vi "Main.vi"() -> ()   [LabVIEW 2020]
uses:
  Archiv/2022-07-15 Labview Burst Preassure Measuring System_neu/Computer/Controls/IMAQdx.ctl
  Controls/SM_UserInterface.ctl
  Controls/SM_DataLog.ctl
  <vilib>/Platform/TimedLoop/XDataNode/timing_clust.ctl
  <vilib>/Platform/TimedLoop/XDataNode/nitl_modes.ctl
  <vilib>/Platform/TimedLoop/XDataNode/wakeup.ctl
  <vilib>/Analysis/baseanly.llb/Mean (DBL).vi
  <vilib>/platform/TimedLoop/XDataNode/XDataNode.xnode
  <vilib>/ptbypt/NI_PtbyPt.lvlib
  <vilib>/Platform/TimedLoop/XDataNode/XDNodeRunTimeDep.lvlib
  Library/Data Buffer.lvlib
  <vilib>/Analysis/NI_AALBase.lvlib
panel:
  in  "OK Exp 2":bool
  in  "Experiment Comment":string
  in  "Buffer Cam4":T1
  in  "Buffer Cam3":T1
  in  "Buffer Cam2":T1
  in  "Buffer Cam1":T1
  out "LoopTimer Cam3":T2
  out "WriteSpeed Cam3":T3 {"WriteSpeed Worker5" format="%_19f"; "WriteSpeed Worker4" format="%_19f"; "WriteSpeed Worker3" format="%_19f"; "WriteSpeed Worker2" format="%_19f"; "WriteSpeed Worker1" format="%_19f"}
  out "Frames Cam3":T4
  out "LoopTimer Cam4":T2
  out "WriteSpeed Cam4":T3 {"WriteSpeed Worker5" format="%_19f"; "WriteSpeed Worker4" format="%_19f"; "WriteSpeed Worker3" format="%_19f"; "WriteSpeed Worker2" format="%_19f"; "WriteSpeed Worker1" format="%_19f"}
  out "Frames Cam4":T4
  out "LoopTimer Cam2":T2
  out "WriteSpeed Cam2":T3 {"WriteSpeed Worker5" format="%_19f"; "WriteSpeed Worker4" format="%_19f"; "WriteSpeed Worker3" format="%_19f"; "WriteSpeed Worker2" format="%_19f"; "WriteSpeed Worker1" format="%_19f"}
  out "Frames Cam2":T4
  out "Frames Cam1":T4
  out "WriteSpeed Cam1":T3 {"WriteSpeed Worker5" format="%_19f"; "WriteSpeed Worker4" format="%_19f"; "WriteSpeed Worker3" format="%_19f"; "WriteSpeed Worker2" format="%_19f"; "WriteSpeed Worker1" format="%_19f"}
  out "LoopTimer Cam1":T2
  in  "Developer":bool
  out "DataFile":bool
  out "Cam4 Time":string
  out "Cam3 Time":string
  out "Cam2 Time":string
  out "Cam1 Time":string
  in  "OK Exp":bool
  out "Stop":bool
  in  "Experiment Comment":string
  in  "Flow Rate Level":i32 min=0 max=99 step=1
  out "IncLoop DataLog":i32
  out "Pressure (mmHg)":dbl format="%.1f"
  out "Waveform Pressure Cluster":waveform(dbl)[](graph)
  out "meanPressureArray":dbl[](array[numeric])
  out "meanPressure":dbl format="%0.2f"
  out "Camera 4":T5(plugin-control)
  out "StartPressure (mmHg)":dbl format="%.2f"
  out "LogFolder":path
  out "StateDataLog":T6
  out "StateUI":T7
  out "CamInput":bool
  out "Start_DateTime":string
  out "LoopTimer UI":u32
  out "Temp (C)":dbl format="%#.1f"
  out "Waveform Chart Temp":waveform(dbl)(graph)
  out "Status Camera 4":bool
  out "Status Camera 3":bool
  out "Status Camera 2":bool
  out "Status Camera 1":bool
  out "Status Temp. Sensor":bool
  out "Status Pressure Sensor":bool
  in  "User":string
  in  "Experiment Infos":string
  in  "Bursting Mode":string(combo)
  out "ExpTime_ms":i32
  out "ActualTime_ms":i32
  out "Camera 1":T5(plugin-control)
  out "Camera 2":T5(plugin-control)
  out "Camera 3":T5(plugin-control)
  in  "IMAQdxChannel 1":T8="cam0" caption="Camera Channel 1"
  in  "OK Input":bool
  in  "IMAQdxChannel 2":T8="cam0" caption="Camera Channel 2"
  in  "IMAQdxChannel 3":T8="cam0" caption="Camera Channel 3"
  in  "IMAQdxChannel 4":T8="cam0" caption="Camera Channel 4"
  out "Status":string="Video OFF"
  in  "Folder":path=path "C:/Users/Public/Downloads" caption="Select path to store video"
  in  "File Name":string
  in  "OK File":bool
  in  "StartRecord":bool caption="Save Video"
  in  "StopRecord":bool
  out "Pressure Temp (C)":dbl
  out "error out":errorcluster
  in  "Cancel":bool
  # "MRI   TUM"
  # "Burst Pressure Measuring System"
  # "1. Select USB Camera Channel"
  # "Pressure in mmHg"
  # "2. Set the Storage Location & Experiment Data"
  # "Temperature in °C"
  # "3. Video and Data Recording"
  # "Sensor Status"
  # "Set before Start Video"
  # "Set before Start Video"
  # "Set before Start Video"
  # "Set before Start Video"
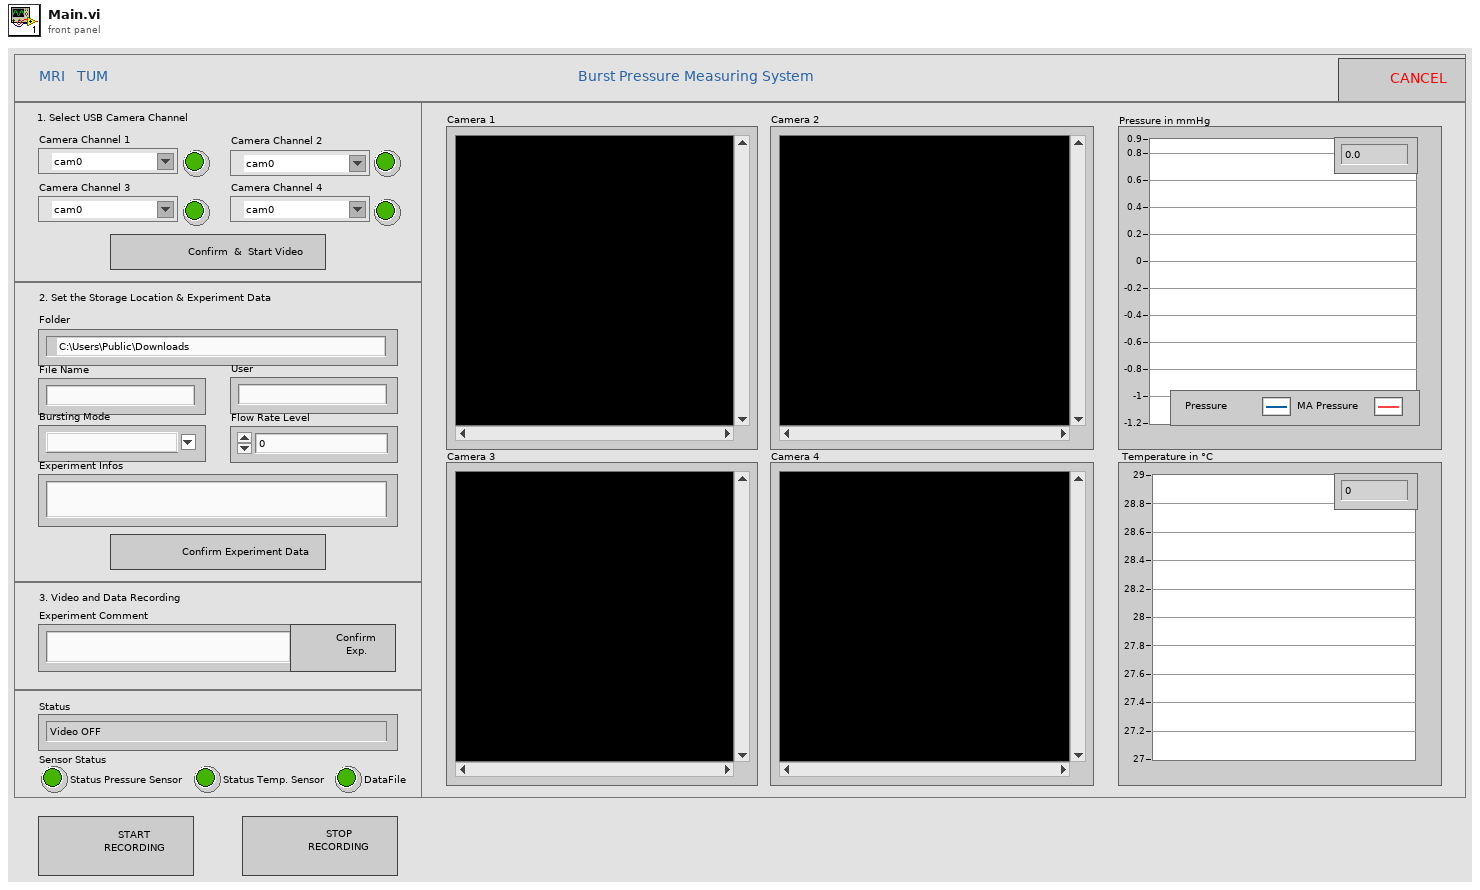
[diagram p1: front panel]
types:
  T1 = cluster{"Skip Count":u32, "Number of Workers":u8, "Number of Images":i32}
  T2 = cluster{"LoopTimerAcqu":u32, "LoopTimer Worker1":u32, "LoopTimer Worker2":u32, "LoopTimer Worker3":u32, "LoopTimer Worker4":u32, "LoopTimer Worker5":u32}
  T3 = cluster{"WriteSpeed Worker1":dbl, "WriteSpeed Worker2":dbl, "WriteSpeed Worker3":dbl, "WriteSpeed Worker4":dbl, "WriteSpeed Worker5":dbl, "Write Speed":dbl}
  T4 = cluster{"Img Processed per Sec":dbl, "Img Behind":i32, "Img Acquired per Sec":dbl}
  T5 = typedef "IMAQ Image.ctl" = refnum<image>
  T6 = typedef "Data Buffer.lvlib/SM_DataLog.ctl" = enum16{"Wait", "CreateFolder", "CreateFile", "WaitRec", "FirstCallWriteData", "WriteData", "LastCallWriteData", "Stop"}
  T7 = typedef "Data Buffer.lvlib/SM_UserInterface.ctl" = enum16{"CamInput", "InitVideo", "InitExpData", "WaitRec", "Recording", "StopRec"}
  T8 = typedef "IMAQdx.ctl" = refnum<k21>
  T9 = enum8{"Enabled", "Disabled", "Disabled and Grayed Out"}
  T10 = typedef "XDNodeRunTimeDep.lvlib/timing_clust.ctl" = cluster{"Expected End [f-1]":u64, "Actual End [f-1]":u64, "Finished Late? [f-1]":bool, "Expected End [i-1]":u64, "Actual End [i-1]":u64, "Finished Late? [i-1]":bool, "Expected Start [i]":u64, "Actual Start [i]":u64, "Expected Start [f]":u64, "Actual Start [f]":u64, "Source Name":string, "Structure Name":string, "Period":i64, "Deadline":i64, "Offset":i64, "Start":i64, "Priority":i32, "Timeout":i32, "Mode":T11, "Wakeup Reason":T12, "Error":errorcluster, "Source Type":string, "Secondary Source Type":string, "Global End Time":u64, "Global Start Time":u64, "Frame Duration":u64, "Iteration Duration":u64, "Assigned CPU":i32, "I/O Scan Engine Mode":u32}
  T11 = typedef "XDNodeRunTimeDep.lvlib/nitl_modes.ctl" = enum32{"No Change", "Process missed periods, maintain original phase", "Discard missed periods, maintain original phase", "Process missed periods, ignore original phase", "Discard missed periods, ignore original phase"}
  T12 = typedef "XDNodeRunTimeDep.lvlib/wakeup.ctl" = enum32{"Normal", "Aborted", "Asynchronous wakeup", "Timing source error", "Timed loop error", "Timeout"}
  T13 = enum16{"open", "replace", "create", "open or create", "replace or create", "replace or create with confirmation"}
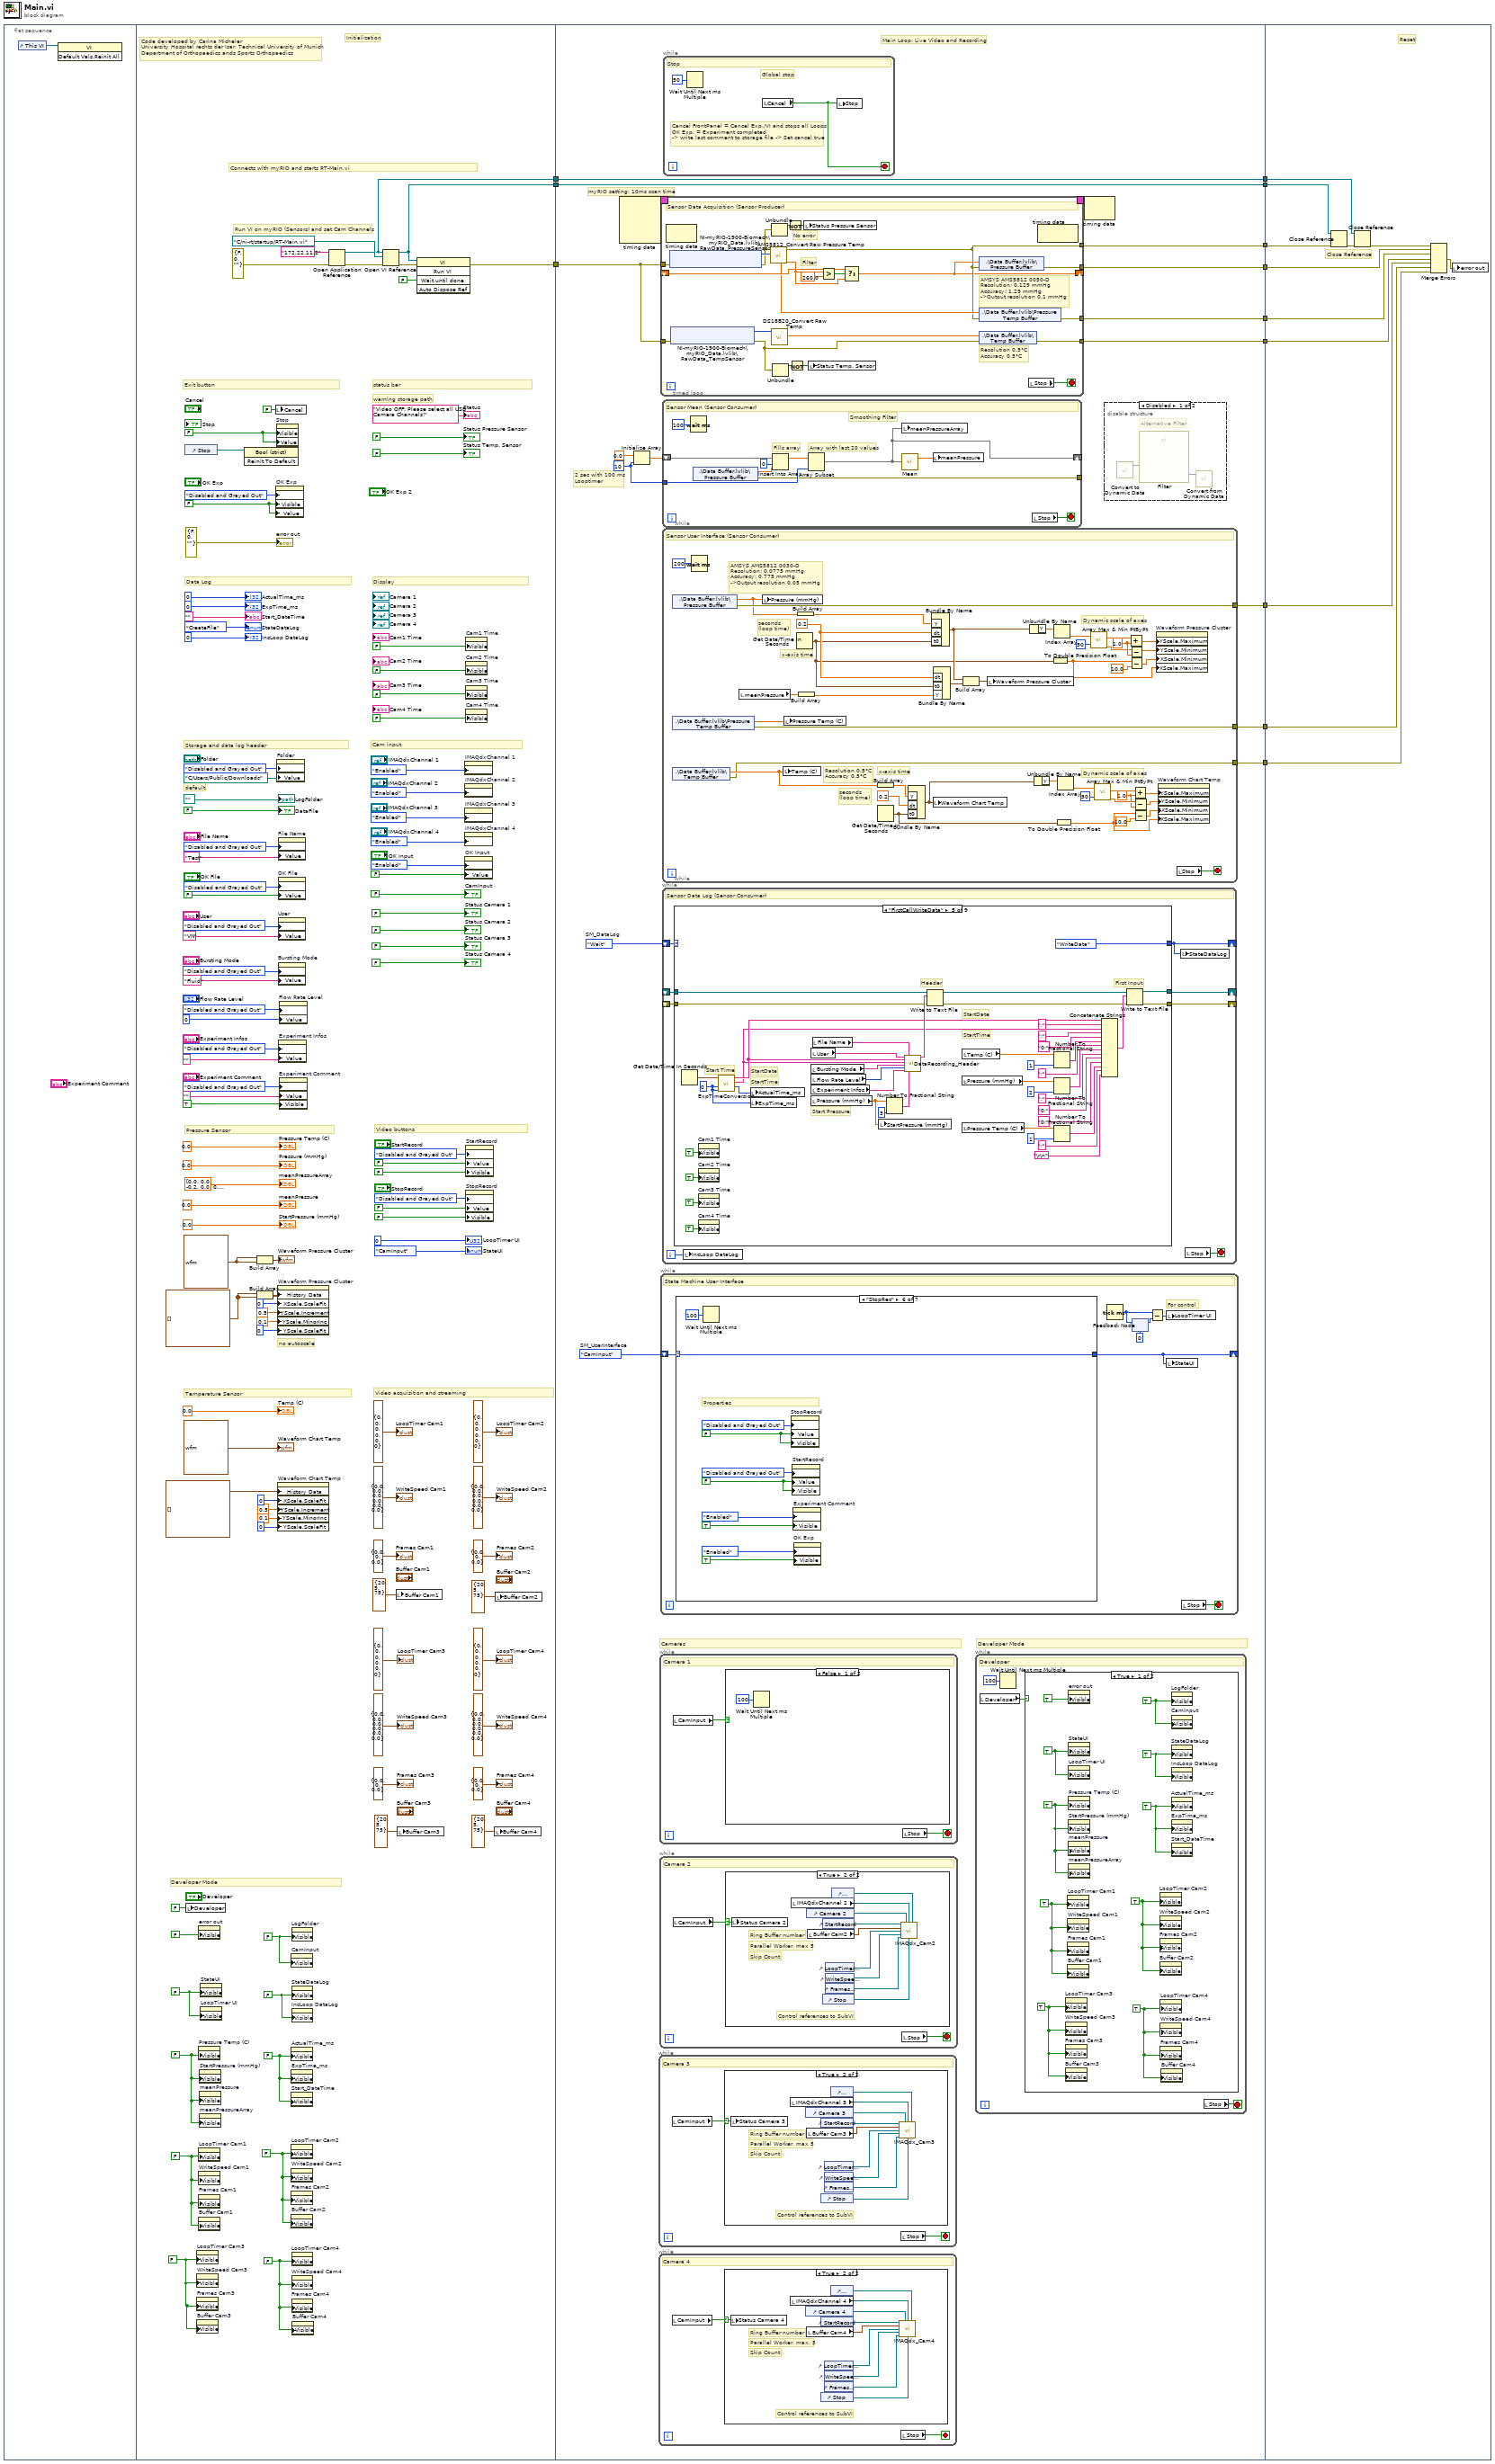
[diagram p0: block diagram]
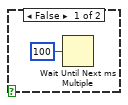
[diagram p3: hidden frame]
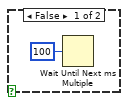
[diagram p4: hidden frame]
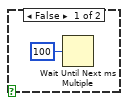
[diagram p5: hidden frame]
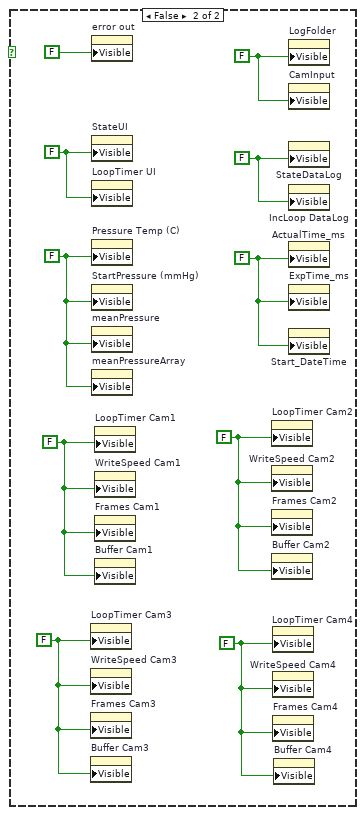
[diagram p6: hidden frame]
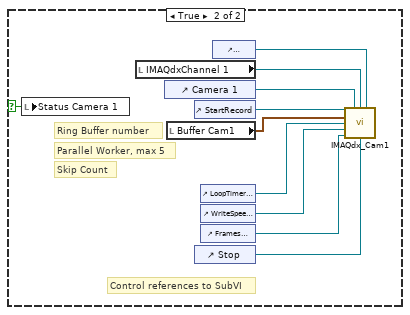
[diagram p7: hidden frame]
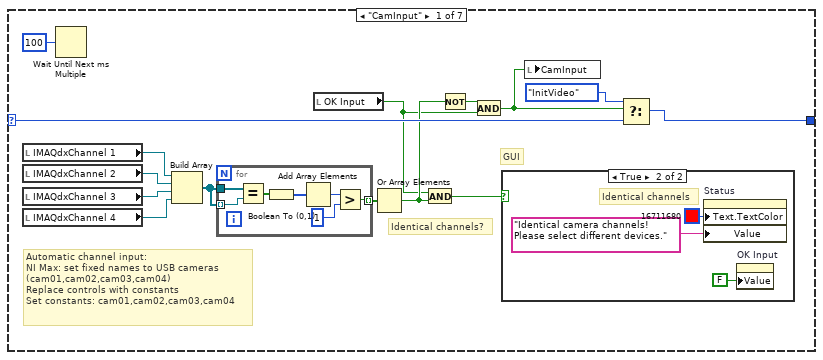
[diagram p8: hidden frame]
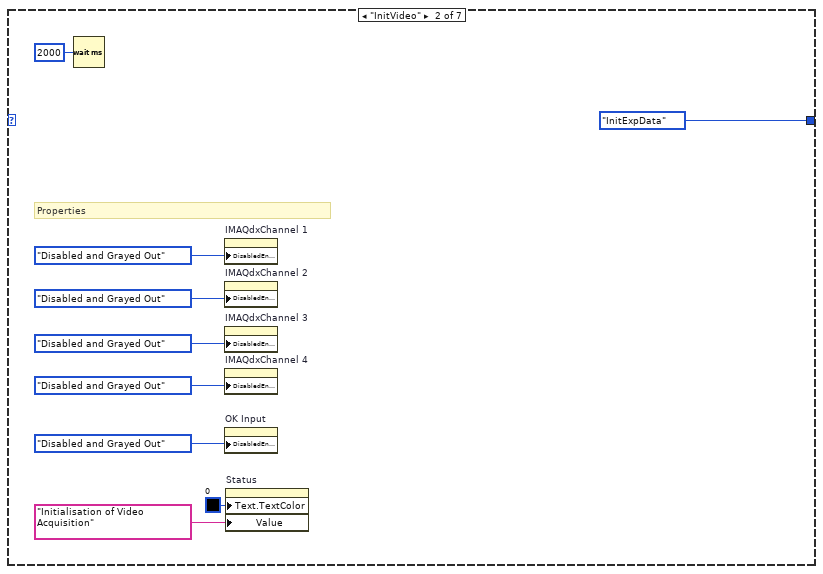
[diagram p10: hidden frame]
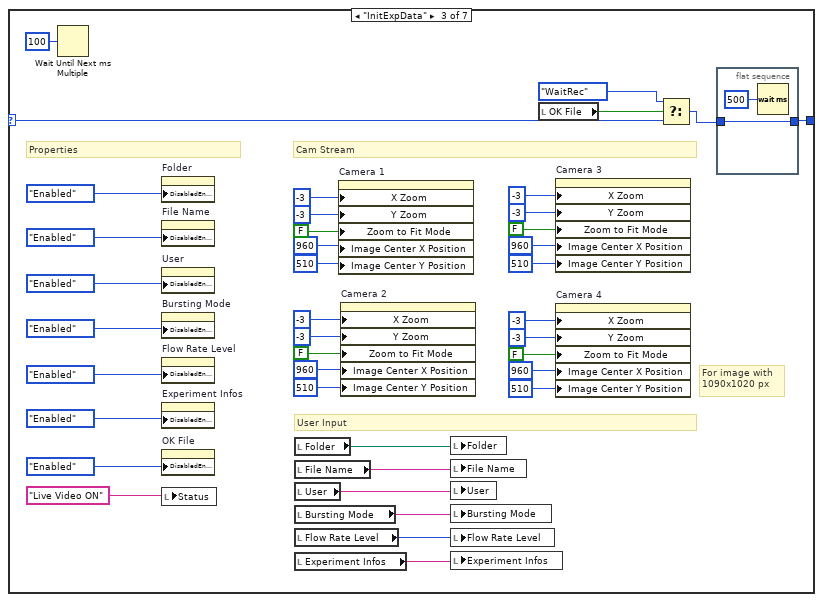
[diagram p11: hidden frame]
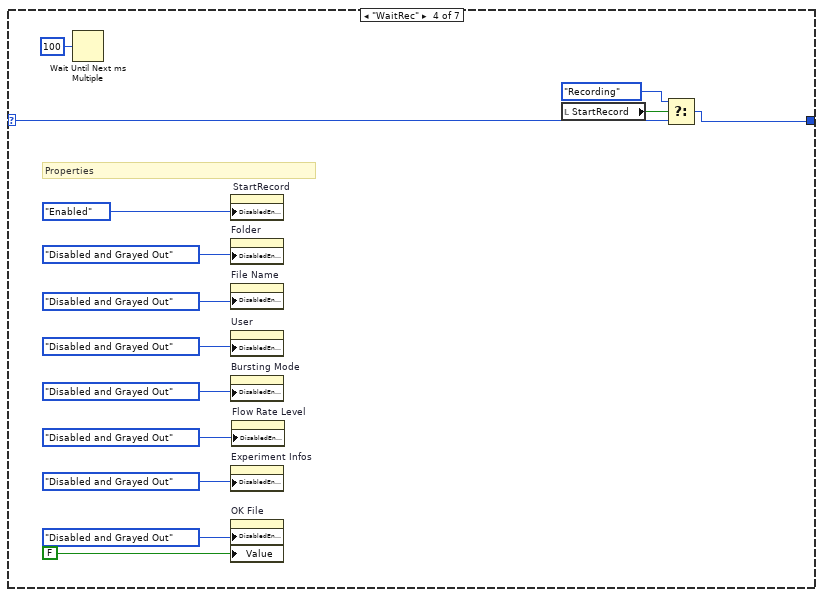
[diagram p12: hidden frame]
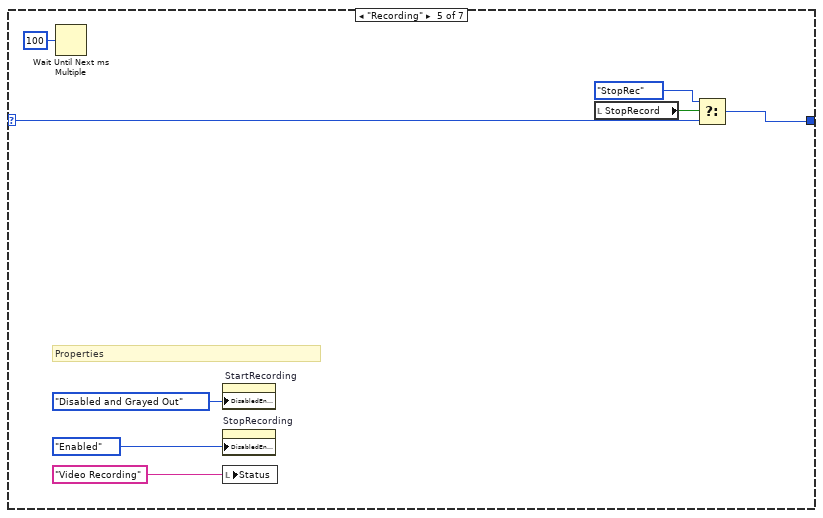
[diagram p13: hidden frame]
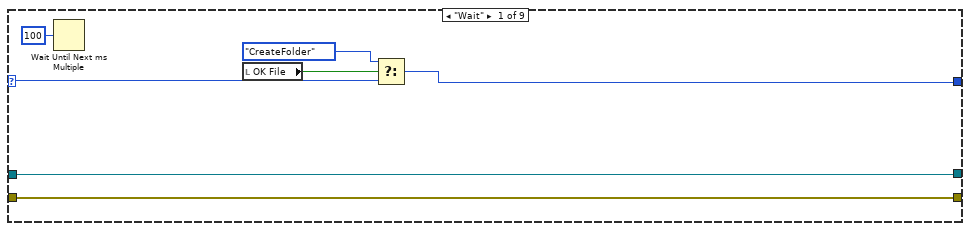
[diagram p15: hidden frame]
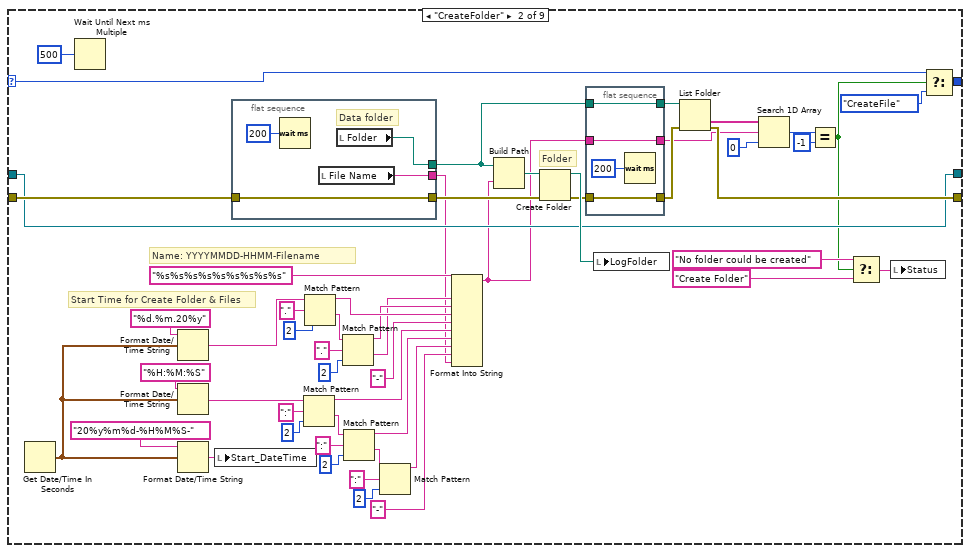
[diagram p16: hidden frame]
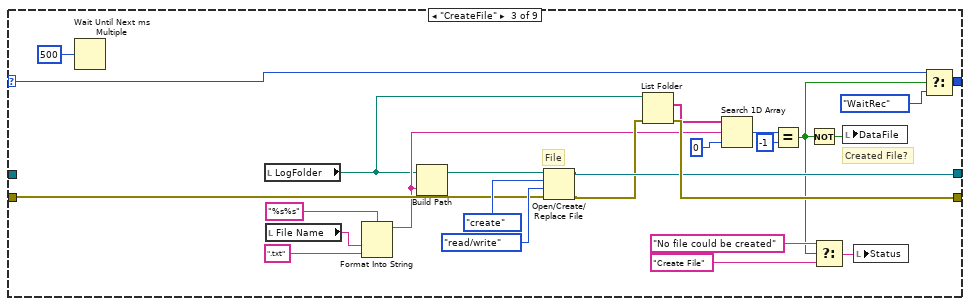
[diagram p17: hidden frame]
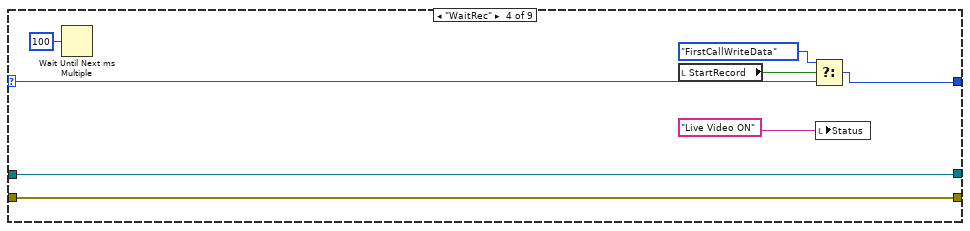
[diagram p18: hidden frame]
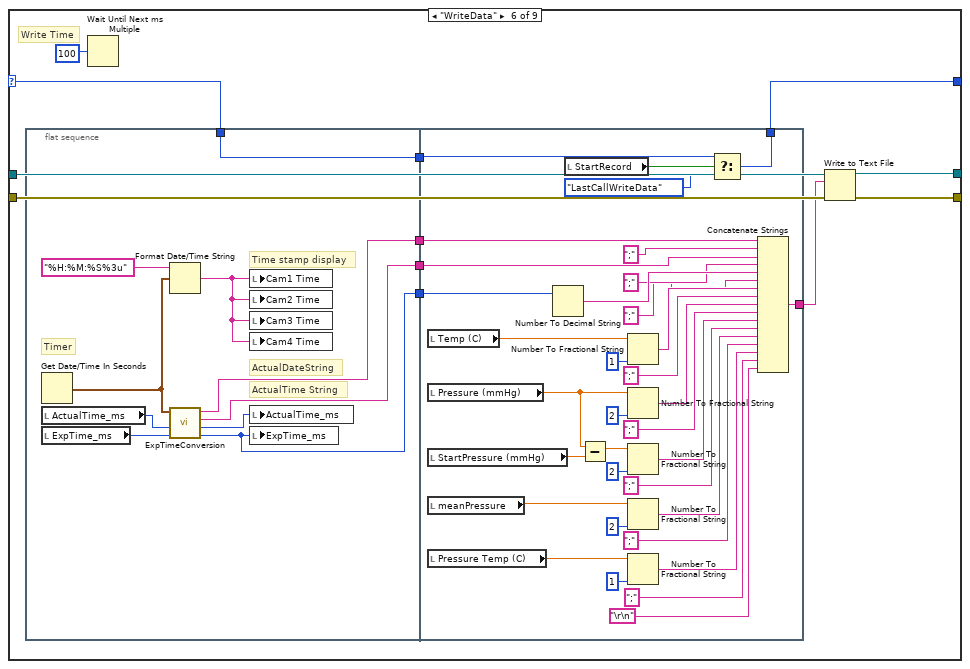
[diagram p19: hidden frame]
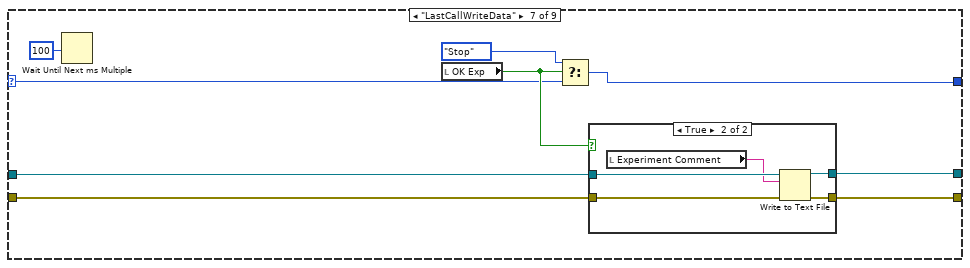
[diagram p20: hidden frame]
diagram:
  n1 = flat-sequence {
    tunnel: [w86] -> w1
    tunnel: [w85] -> w3
    tunnel: [w84] -> w2
    tunnel: [w142] -> w12
    tunnel: [w141] -> w11
    tunnel: w3 -> [w142]
    tunnel: w2 -> [w141]
    tunnel: w1 -> [w126]
    tunnel: [w137] -> w10
    tunnel: [w136] -> w9
    tunnel: [w135] -> w8
    tunnel: [w134] -> w7
    tunnel: [w133] -> w6
    tunnel: [w132] -> w5
    tunnel: [w131] -> w4
    tunnel: w12 -> [w663]
    tunnel: w11 -> [w664]
    tunnel: w10 -> [w660]
    tunnel: w9 -> [w659]
    tunnel: w8 -> [w658]
    tunnel: w7 -> [w657]
    tunnel: w6 -> [w656]
    tunnel: w5 -> [w655]
    tunnel: w4 -> [w654]
    frame #0 {
      n2 = control-ref of="This VI"() -> (w13:refnum<vi>)
      n3 = invoke class="VI" method="Default Vals.Reinit All"(reference=w13) -> ()  [unwired: 2 in, 3 out]
    }
    frame #1 {
      w22 = FALSE ("Visible")
      w23 = FALSE ("Visible")
      w24 = FALSE ("Visible")
      w18 = FALSE ("Visible")
      w21 = FALSE ("Visible")
      w26 = FALSE ("Visible")
      w25 = FALSE ("Visible")
      w19 = FALSE ("Visible")
      w20 = FALSE ("Visible")
      w63 = FALSE ("Visible")
      w66 = FALSE ("Exit")
      w75 = waveform(dbl)[] [] ("History Data")
      w77 = waveform(dbl) {"t0"=timestamp(0 s since 1904-01-01), "dt"=1.0, "Y"=[]} ("Waveform Chart Pressure")
      # "Developer Mode"
      # "Code developed by Carina Micheler\nUniversity Hospital rechts der Isar, Technical University of Munich\nDepartment of Orthopaedics ands Sports Orthopaedics"
      # "Video acquisition and streaming"
      # "Data Log"
      # "Connects with myRIO and starts RT-Main.vi"
      # "Run VI on myRIO (Sensors) and set Cam Channels"
      # "no autoscale"
      # "warning storage path"
      # "status bar"
      # "Video buttons"
      # "default"
      # "Storage and data log header"
      # "Temperature Sensor"
      # "Pressure Sensor"
      # "Display"
      # "Cam input"
      # "Exit button"
      # "Initialization"
      n4 = control-ref of="Stop"() -> (w42:refnum<vi>)
      n5 = local write "Developer"(FALSE ("Developer")) -> ()
      n6 = property on="LoopTimer Cam3" class="Clust (strict)"("Visible"=w19) -> ()  [unwired: 2 in, 2 out]
      n7 = property on="WriteSpeed Cam3" class="Clust (strict)"("Visible"=w19) -> ()  [unwired: 2 in, 2 out]
      n8 = property on="Frames Cam3" class="Clust (strict)"("Visible"=w19) -> ()  [unwired: 2 in, 2 out]
      n9 = property on="Buffer Cam3" class="Clust (strict)"("Visible"=w19) -> ()  [unwired: 2 in, 2 out]
      n10 = property on="error out" class="Clust (strict)"("Visible"=FALSE) -> ()  [unwired: 2 in, 2 out]
      n11 = property on="Pressure Temp (C)" class="DigNum (strict)"("Visible"=w25) -> ()  [unwired: 2 in, 2 out]
      n12 = property on="LoopTimer Cam1" class="Clust (strict)"("Visible"=w20) -> ()  [unwired: 2 in, 2 out]
      n13 = property on="WriteSpeed Cam1" class="Clust (strict)"("Visible"=w20) -> ()  [unwired: 2 in, 2 out]
      n14 = property on="Frames Cam1" class="Clust (strict)"("Visible"=w20) -> ()  [unwired: 2 in, 2 out]
      n15 = property on="Buffer Cam1" class="Clust (strict)"("Visible"=w20) -> ()  [unwired: 2 in, 2 out]
      n16 = property on="StartPressure (mmHg)" class="DigNum (strict)"("Visible"=w25) -> ()  [unwired: 2 in, 2 out]
      n17 = property on="meanPressure" class="DigNum (strict)"("Visible"=w25) -> ()  [unwired: 2 in, 2 out]
      n18 = property on="meanPressureArray" class="Arr (strict)"("Visible"=w25) -> ()  [unwired: 2 in, 2 out]
      n19 = property on="StateUI" class="Enum (strict)"("Visible"=w23) -> ()  [unwired: 2 in, 2 out]
      n20 = property on="LoopTimer UI" class="DigNum (strict)"("Visible"=w23) -> ()  [unwired: 2 in, 2 out]
      n21 = invoke class="Bool (strict)" method="Reinit To Default"(reference=w42) -> ()  [unwired: 2 in, 3 out]
      n22 = Build Array(w77, w77) -> (→"Waveform Pressure Cluster":waveform(dbl)[])
      n23 = Build Array(w75, w75) -> (w76:waveform(dbl)[][])
      n24 = local write "Cancel"(FALSE ("Cancel")) -> ()
      n25 = property on="OK Exp" class="Bool (strict)"("DisabledEnum"=T9."Disabled and Grayed Out" ("Disabled"), "Visible"=w63, "Value"=w63) -> ()  [unwired: 2 in, 2 out]
      n26 = property on="Stop" class="Bool (strict)"("Visible"=w66, "Value"=w66) -> ()  [unwired: 2 in, 2 out]
      n27 = property on="Folder" class="Path"("DisabledEnum"=T9."Disabled and Grayed Out" ("Disabled"), "Value"=path "C:/Users/Public/Downloads" ("VideoFolder")) -> ()  [unwired: 2 in, 2 out]
      n28 = property on="Waveform Pressure Cluster" class="WFChart (strict)"("History Data"=w76, "XScale.ScaleFit"=u8 0 ("X Scale.Scale Fit"), "YScale.Increment"=0.5 ("Y Scale.Range:Increment"), "YScale.MinorInc"=0.1 ("Y Scale.Range:Minor Increment"), "YScale.ScaleFit"=u8 0 ("Y Scale.Scale Fit")) -> ()  [unwired: 2 in, 2 out]
      n29 = property on="Waveform Chart Temp" class="WFChart (strict)"("History Data"=waveform(dbl)[] [], "XScale.ScaleFit"=u8 0 ("X Scale.Scale Fit"), "YScale.Increment"=0.5 ("Y Scale.Range:Increment"), "YScale.MinorInc"=0.1 ("Y Scale.Range:Minor Increment"), "YScale.ScaleFit"=u8 0 ("Y Scale.Scale Fit")) -> ()  [unwired: 2 in, 2 out]
      n30 = property on="File Name" class="Str"("DisabledEnum"=T9."Disabled and Grayed Out" ("Disabled"), "Value"="Test" ("Name")) -> ()  [unwired: 2 in, 2 out]
      n31 = property on="OK File" class="Bool (strict)"("DisabledEnum"=T9."Disabled and Grayed Out" ("Disabled"), "Value"=FALSE ("OK Button File")) -> ()  [unwired: 2 in, 2 out]
      n32 = property on="User" class="Str"("DisabledEnum"=T9."Disabled and Grayed Out" ("Disabled"), "Value"="VN" ("Name")) -> ()  [unwired: 2 in, 2 out]
      n33 = property on="Bursting Mode" class="CmbBox"("DisabledEnum"=T9."Disabled and Grayed Out" ("Disabled"), "Value"="Fluid" ("Name")) -> ()  [unwired: 2 in, 2 out]
      n34 = property on="Experiment Infos" class="Str"("DisabledEnum"=T9."Disabled and Grayed Out" ("Disabled"), "Value"="" ("Name")) -> ()  [unwired: 2 in, 2 out]
      n35 = property on="Flow Rate Level" class="DigNum (strict)"("DisabledEnum"=T9."Disabled and Grayed Out" ("Disabled"), "Value"=0 ("Flow Rate Level")) -> ()  [unwired: 2 in, 2 out]
      n36 = property on="Experiment Comment" class="Str"("DisabledEnum"=T9."Disabled and Grayed Out" ("Disabled"), "Value"="" ("Experiment Comment"), "Visible"=TRUE) -> ()  [unwired: 2 in, 2 out]
      n37 = property on="CamInput" class="Bool (strict)"("Visible"=w24) -> ()  [unwired: 2 in, 2 out]
      n38 = property on="ActualTime_ms" class="DigNum (strict)"("Visible"=w26) -> ()  [unwired: 2 in, 2 out]
      n39 = property on="ExpTime_ms" class="DigNum (strict)"("Visible"=w26) -> ()  [unwired: 2 in, 2 out]
      n40 = property on="Start_DateTime" class="Str"("Visible"=w26) -> ()  [unwired: 2 in, 2 out]
      n41 = property on="LoopTimer Cam2" class="Clust (strict)"("Visible"=w21) -> ()  [unwired: 2 in, 2 out]
      n42 = property on="WriteSpeed Cam2" class="Clust (strict)"("Visible"=w21) -> ()  [unwired: 2 in, 2 out]
      n43 = property on="Frames Cam2" class="Clust (strict)"("Visible"=w21) -> ()  [unwired: 2 in, 2 out]
      n44 = property on="Buffer Cam2" class="Clust (strict)"("Visible"=w21) -> ()  [unwired: 2 in, 2 out]
      n45 = property on="LogFolder" class="Path"("Visible"=w24) -> ()  [unwired: 2 in, 2 out]
      n46 = property on="StateDataLog" class="Enum (strict)"("Visible"=w22) -> ()  [unwired: 2 in, 2 out]
      n47 = property on="IncLoop DataLog" class="DigNum (strict)"("Visible"=w22) -> ()  [unwired: 2 in, 2 out]
      n48 = property on="LoopTimer Cam4" class="Clust (strict)"("Visible"=w18) -> ()  [unwired: 2 in, 2 out]
      n49 = property on="WriteSpeed Cam4" class="Clust (strict)"("Visible"=w18) -> ()  [unwired: 2 in, 2 out]
      n50 = property on="Frames Cam4" class="Clust (strict)"("Visible"=w18) -> ()  [unwired: 2 in, 2 out]
      n51 = property on="Buffer Cam4" class="Clust (strict)"("Visible"=w18) -> ()  [unwired: 2 in, 2 out]
      n52 = Open Application Reference(8:errorcluster {"status"=FALSE, "code"=0, "source"=""} ("error in (no error)"), 11:"172.22.11.2" ("machine name (\"\":  open local reference)")) -> (0:w92:errorcluster, 3:w84:refnum<vi>)  [unwired: 2 in]
      n53 = Open VI Reference(application reference (local)=w84, vi path=path "C:/ni-rt/startup/RT-Main.vi", error in (no error)=w92) -> (vi reference=w85:refnum<vi>, error out=w91:errorcluster)  [unwired: 3 in]
      n54 = local write "Buffer Cam1"(T1 {"Skip Count"=20, "Number of Workers"=5, "Number of Images"=75} ("Buffer Cam1")) -> ()
      n55 = local write "Buffer Cam3"(T1 {"Skip Count"=20, "Number of Workers"=5, "Number of Images"=75} ("Buffer Cam3")) -> ()
      n56 = invoke class="VI" method="Run VI"(reference=w85, error in=w91, "Wait until done"=FALSE ("Wait Until Done")) -> (error out=w86:errorcluster)  [unwired: 2 in, 4 out]
      n57 = property on="IMAQdxChannel 1" class="IMAQdx (strict)"("DisabledEnum"=T9."Enabled" ("Disabled")) -> ()  [unwired: 2 in, 2 out]
      n58 = property on="IMAQdxChannel 2" class="IMAQdx (strict)"("DisabledEnum"=T9."Enabled" ("Disabled")) -> ()  [unwired: 2 in, 2 out]
      n59 = property on="IMAQdxChannel 3" class="IMAQdx (strict)"("DisabledEnum"=T9."Enabled" ("Disabled")) -> ()  [unwired: 2 in, 2 out]
      n60 = property on="IMAQdxChannel 4" class="IMAQdx (strict)"("DisabledEnum"=T9."Enabled" ("Disabled")) -> ()  [unwired: 2 in, 2 out]
      n61 = property on="OK Input" class="Bool (strict)"("DisabledEnum"=T9."Enabled" ("Disabled"), "Value"=FALSE ("OK Button")) -> ()  [unwired: 2 in, 2 out]
      n62 = property on="Cam1 Time" class="Str"("Visible"=FALSE) -> ()  [unwired: 2 in, 2 out]
      n63 = property on="Cam2 Time" class="Str"("Visible"=FALSE) -> ()  [unwired: 2 in, 2 out]
      n64 = property on="Cam3 Time" class="Str"("Visible"=FALSE) -> ()  [unwired: 2 in, 2 out]
      n65 = property on="Cam4 Time" class="Str"("Visible"=FALSE) -> ()  [unwired: 2 in, 2 out]
      n66 = property on="StartRecord" class="Bool (strict)"("DisabledEnum"=T9."Disabled and Grayed Out" ("Disabled"), "Value"=FALSE ("StartRecord"), "Visible"=FALSE) -> ()  [unwired: 2 in, 2 out]
      n67 = property on="StopRecord" class="Bool (strict)"("DisabledEnum"=T9."Disabled and Grayed Out" ("Disabled"), "Value"=FALSE ("StopRecord"), "Visible"=FALSE) -> ()  [unwired: 2 in, 2 out]
      n68 = local write "Buffer Cam4"(T1 {"Skip Count"=20, "Number of Workers"=5, "Number of Images"=75} ("Buffer Cam4")) -> ()
      n69 = local write "Buffer Cam2"(T1 {"Skip Count"=20, "Number of Workers"=5, "Number of Images"=75} ("Buffer Cam2")) -> ()
      "Temp (C)" <- 0.0 ("Temp (C)")
      "Pressure (mmHg)" <- 0.0 ("Pressure (mmHg)")
      "Pressure Temp (C)" <- 0.0 ("Pressure Temp (C)")
      "Status" <- "Video OFF: Please select all USB Camera Channels!" ("Warning 2")
      "ActualTime_ms" <- 0 ("ActualTime_ms")
      "ExpTime_ms" <- 0 ("ExpTime_ms")
      "error out" <- errorcluster {"status"=FALSE, "code"=0, "source"=""} ("error out")
      "Status Temp. Sensor" <- FALSE ("State Temp. Sensor")
      "Status Pressure Sensor" <- FALSE ("State Pressure Sensor")
      "Status Camera 3" <- FALSE ("Camera 3")
      "Status Camera 4" <- FALSE ("Camera 4")
      "Status Camera 1" <- FALSE ("Camera 1")
      "Status Camera 2" <- FALSE ("Camera 2")
      "Waveform Chart Temp" <- waveform(dbl) {"t0"=timestamp(0 s since 1904-01-01), "dt"=1.0, "Y"=[]} ("Waveform Chart Temp")
      "CamInput" <- FALSE ("CamInput")
      "StateUI" <- SM_UserInterface."CamInput" ("StateUI")
      "Start_DateTime" <- "" ("Start_DateTime")
      "StateDataLog" <- SM_DataLog."CreateFile" ("StateDataLog")
      "StartPressure (mmHg)" <- 0.0 ("StartPressure (mmHg)")
      "meanPressure" <- 0.0 ("meanPressure")
      "meanPressureArray" <- dbl[] [0.0, 0.0, -0.2, 0.0, 0.0, 0.0, 0.0, 0.0, 0.0, 0.0, 0.0, 0.0, 0.0, 0.0, 0.0, -0.2, 0.0, 0.0, 0.0, 0.0] ("meanPressureArray")
      "LogFolder" <- path "" ("LogFolder")
      "LoopTimer UI" <- u32 0 ("LoopTimer UI")
      "IncLoop DataLog" <- 0 ("IncLoop DataLog")
      "DataFile" <- FALSE ("DataLog")
      "LoopTimer Cam1" <- T2 {"LoopTimerAcqu"=0, "LoopTimer Worker1"=0, "LoopTimer Worker2"=0, "LoopTimer Worker3"=0, "LoopTimer Worker4"=0, "LoopTimer Worker5"=0} ("Cluster LoopTimer")
      "WriteSpeed Cam1" <- T3 {"WriteSpeed Worker1"=0.0, "WriteSpeed Worker2"=0.0, "WriteSpeed Worker3"=0.0, "WriteSpeed Worker4"=0.0, "WriteSpeed Worker5"=0.0, "Write Speed"=0.0} ("Cluster WriteSpeed")
      "Frames Cam1" <- T4 {"Img Processed per Sec"=0.0, "Img Behind"=0, "Img Acquired per Sec"=0.0} ("Cluster Frames")
      "LoopTimer Cam2" <- T2 {"LoopTimerAcqu"=0, "LoopTimer Worker1"=0, "LoopTimer Worker2"=0, "LoopTimer Worker3"=0, "LoopTimer Worker4"=0, "LoopTimer Worker5"=0} ("Cluster LoopTimer")
      "WriteSpeed Cam2" <- T3 {"WriteSpeed Worker1"=0.0, "WriteSpeed Worker2"=0.0, "WriteSpeed Worker3"=0.0, "WriteSpeed Worker4"=0.0, "WriteSpeed Worker5"=0.0, "Write Speed"=0.0} ("Cluster WriteSpeed")
      "Frames Cam2" <- T4 {"Img Processed per Sec"=0.0, "Img Behind"=0, "Img Acquired per Sec"=0.0} ("Cluster Frames")
      "LoopTimer Cam3" <- T2 {"LoopTimerAcqu"=0, "LoopTimer Worker1"=0, "LoopTimer Worker2"=0, "LoopTimer Worker3"=0, "LoopTimer Worker4"=0, "LoopTimer Worker5"=0} ("Cluster LoopTimer")
      "WriteSpeed Cam3" <- T3 {"WriteSpeed Worker1"=0.0, "WriteSpeed Worker2"=0.0, "WriteSpeed Worker3"=0.0, "WriteSpeed Worker4"=0.0, "WriteSpeed Worker5"=0.0, "Write Speed"=0.0} ("Cluster WriteSpeed")
      "Frames Cam3" <- T4 {"Img Processed per Sec"=0.0, "Img Behind"=0, "Img Acquired per Sec"=0.0} ("Cluster Frames")
      "LoopTimer Cam4" <- T2 {"LoopTimerAcqu"=0, "LoopTimer Worker1"=0, "LoopTimer Worker2"=0, "LoopTimer Worker3"=0, "LoopTimer Worker4"=0, "LoopTimer Worker5"=0} ("Cluster LoopTimer")
      "WriteSpeed Cam4" <- T3 {"WriteSpeed Worker1"=0.0, "WriteSpeed Worker2"=0.0, "WriteSpeed Worker3"=0.0, "WriteSpeed Worker4"=0.0, "WriteSpeed Worker5"=0.0, "Write Speed"=0.0} ("Cluster WriteSpeed")
      "Frames Cam4" <- T4 {"Img Processed per Sec"=0.0, "Img Behind"=0, "Img Acquired per Sec"=0.0} ("Cluster Frames")
    }
    frame #2 {
      w127 = 10 ("dimension size")
      w130 = SM_UserInterface."CamInput"  # SM_UserInterface
      w140 = SM_DataLog."Wait"  # SM_DataLog
      # "Developer Mode"
      # "Cameras"
      # "2 sec with 100 ms\nLooptimer"
      # "myRIO setting: 10ms scan time"
      # "Main Loop: Live Video and Recording"
      n70 = node-c288() -> (w139:T10)  [unwired: 4 in]
      n71 = Initialize Array(0.0 ("element"), w127) -> (w128:dbl[])
      n72 = while {
        stop <- w158 stop-if-true
        # "Camera 3"
        n73 = local read "CamInput"() -> (w159:bool)
        n74 = case shown="True" w159 {
          selector: w159 -> [_ w161]
          frame False {
            n75 = Wait Until Next ms Multiple(millisecond multiple=u32 100) -> ()  [unwired: 1 out]
          }
          frame True {
            # "Control references to SubVI"
            # "Parallel Worker, max 5"
            # "Skip Count"
            # "Ring Buffer number"
            n76 = local write "Status Camera 3"(w161) -> ()
            n77 = local read "IMAQdxChannel 3"() -> (w170:T8)
            n78 = control-ref of="Camera 3"() -> (w167:refnum<vi>)
            n79 = local read "Buffer Cam3"() -> (w162:T1)
            n80 = control-ref of="StartRecord"() -> (w169:refnum<vi>)
            n81 = control-ref of="Stop"() -> (w168:refnum<vi>)
            n82 = control-ref of="LoopTimer Cam3"() -> (w166:refnum<vi>)
            n83 = control-ref of="WriteSpeed Cam3"() -> (w165:refnum<vi>)
            n84 = control-ref of="Frames Cam3"() -> (w164:refnum<vi>)
            n85 = control-ref of="LogFolder"() -> (w163:refnum<vi>)
            n86 = call "IMAQdx_Cam3.vi"("Ctl Ref Record"=w169, "Ctl Ref Cam"=w167, "Session In"=w170, "Ctl Ref Folder"=w163, "Cluster Buffer"=w162, "Ctl Ref Time"=w166, "Ctl Ref WriteSpeed"=w165, "Ctl Ref Frames"=w164, "Ctl Ref Stop"=w168) -> ()  [unwired: 7 in]
          }
        }
        n87 = local read "Stop"() -> (w158:bool)
      }
      n88 = while {
        stop <- w145 stop-if-true
        # "Camera 4"
        n89 = local read "CamInput"() -> (w146:bool)
        n90 = case shown="True" w146 {
          selector: w146 -> [_ w148]
          frame False {
            n91 = Wait Until Next ms Multiple(millisecond multiple=u32 100) -> ()  [unwired: 1 out]
          }
          frame True {
            # "Control references to SubVI"
            # "Parallel Worker, max. 5"
            # "Skip Count"
            # "Ring Buffer number"
            n92 = local write "Status Camera 4"(w148) -> ()
            n93 = local read "IMAQdxChannel 4"() -> (w157:T8)
            n94 = control-ref of="Camera 4"() -> (w151:refnum<vi>)
            n95 = local read "Buffer Cam4"() -> (w149:T1)
            n96 = control-ref of="StartRecord"() -> (w156:refnum<vi>)
            n97 = control-ref of="Stop"() -> (w155:refnum<vi>)
            n98 = control-ref of="LoopTimer Cam4"() -> (w152:refnum<vi>)
            n99 = control-ref of="WriteSpeed Cam4"() -> (w153:refnum<vi>)
            n100 = control-ref of="Frames Cam4"() -> (w154:refnum<vi>)
            n101 = control-ref of="LogFolder"() -> (w150:refnum<vi>)
            n102 = call "IMAQdx_Cam4.vi"("Ctl Ref Record"=w156, "Ctl Ref Cam"=w151, "Session In"=w157, "Ctl Ref Folder"=w150, "Cluster Buffer"=w149, "Ctl Ref Time"=w152, "Ctl Ref WriteSpeed"=w153, "Ctl Ref Frames"=w154, "Ctl Ref Stop"=w155) -> ()  [unwired: 7 in]
          }
        }
        n103 = local read "Stop"() -> (w145:bool)
      }
      n104 = while {
        stop <- w207 stop-if-true
        # "Camera 1"
        n105 = local read "CamInput"() -> (w208:bool)
        n106 = case shown="False" w208 {
          selector: w208 -> [_ w210]
          frame False {
            n107 = Wait Until Next ms Multiple(millisecond multiple=u32 100) -> ()  [unwired: 1 out]
          }
          frame True {
            # "Control references to SubVI"
            # "Parallel Worker, max 5"
            # "Skip Count"
            # "Ring Buffer number"
            n108 = local write "Status Camera 1"(w210) -> ()
            n109 = local read "IMAQdxChannel 1"() -> (w219:T8)
            n110 = control-ref of="Camera 1"() -> (w218:refnum<vi>)
            n111 = local read "Buffer Cam1"() -> (w211:T1)
            n112 = control-ref of="StartRecord"() -> (w217:refnum<vi>)
            n113 = control-ref of="Stop"() -> (w215:refnum<vi>)
            n114 = control-ref of="LoopTimer Cam1"() -> (w216:refnum<vi>)
            n115 = control-ref of="WriteSpeed Cam1"() -> (w214:refnum<vi>)
            n116 = control-ref of="Frames Cam1"() -> (w213:refnum<vi>)
            n117 = control-ref of="LogFolder"() -> (w212:refnum<vi>)
            n118 = call "IMAQdx_Cam1.vi"("Ctl Ref Record"=w217, "Ctl Ref Cam"=w218, "Session In"=w219, "Ctl Ref Folder"=w212, "Cluster Buffer"=w211, "Ctl Ref Time"=w216, "Ctl Ref WriteSpeed"=w214, "Ctl Ref Frames"=w213, "Ctl Ref Stop"=w215) -> ()  [unwired: 7 in]
          }
        }
        n119 = local read "Stop"() -> (w207:bool)
      }
      n120 = while {
        stop <- w171 stop-if-true
        # "Camera 2"
        n121 = local read "CamInput"() -> (w172:bool)
        n122 = case shown="True" w172 {
          selector: w172 -> [_ w174]
          frame False {
            n123 = Wait Until Next ms Multiple(millisecond multiple=u32 100) -> ()  [unwired: 1 out]
          }
          frame True {
            # "Control references to SubVI"
            # "Parallel Worker, max 5"
            # "Skip Count"
            # "Ring Buffer number"
            n124 = local write "Status Camera 2"(w174) -> ()
            n125 = local read "IMAQdxChannel 2"() -> (w183:T8)
            n126 = control-ref of="Camera 2"() -> (w180:refnum<vi>)
            n127 = local read "Buffer Cam2"() -> (w175:T1)
            n128 = control-ref of="StartRecord"() -> (w182:refnum<vi>)
            n129 = control-ref of="Stop"() -> (w181:refnum<vi>)
            n130 = control-ref of="LoopTimer Cam2"() -> (w177:refnum<vi>)
            n131 = control-ref of="WriteSpeed Cam2"() -> (w178:refnum<vi>)
            n132 = control-ref of="Frames Cam2"() -> (w179:refnum<vi>)
            n133 = control-ref of="LogFolder"() -> (w176:refnum<vi>)
            n134 = call "IMAQdx_Cam2.vi"("Ctl Ref Record"=w182, "Ctl Ref Cam"=w180, "Session In"=w183, "Ctl Ref Folder"=w176, "Cluster Buffer"=w175, "Ctl Ref Time"=w177, "Ctl Ref WriteSpeed"=w178, "Ctl Ref Frames"=w179, "Ctl Ref Stop"=w181) -> ()  [unwired: 7 in]
          }
        }
        n135 = local read "Stop"() -> (w171:bool)
      }
      n136 = while {
        shift-right: [w234] -> _
        shift-left: w130 -> [w238]
        stop <- w232 stop-if-true
        # "For control"
        # "State Machine User Interface"
        n137 = case shown="\"StopRec\"" w238 {
          selector: w238 -> [w252 _ w307 w317 w336 w338 w347]
          tunnel: [w250 SM_UserInterface."InitExpData" w273 w328 w335 w338 w347] -> w234
          frame "CamInput" {
            # "Automatic channel input:\nNI Max: set fixed names to USB cameras\n(cam01,cam02,cam03,cam04)\nReplace controls with constants\nSet constants: cam01,cam02,cam03,cam04"
            # "GUI"
            # "Identical channels?"
            n138 = local read "IMAQdxChannel 1"() -> (w246:T8)
            n139 = local read "IMAQdxChannel 2"() -> (w247:T8)
            n140 = local read "IMAQdxChannel 3"() -> (w249:T8)
            n141 = local read "IMAQdxChannel 4"() -> (w248:T8)
            n142 = Wait Until Next ms Multiple(millisecond multiple=u32 100) -> ()  [unwired: 1 out]
            n143 = Build Array(w246, w247, w249, w248) -> (w245:T8[])
            n144 = for {
              tunnel: w245 -> [w263]
              tunnel: w245 -> [w262] mode=indexing
              tunnel: [w258] -> w244 mode=indexing
              n145 = Equal?(x=w263, y=w262) -> (x = y?=w261:bool[])
              n146 = Boolean To (0,1)(Boolean=w261) -> (0, 1=w260:i16[])
              n147 = Add Array Elements(numeric array=w260) -> (sum=w257:i16)
              n148 = Greater?(x=w257, y=i16 1) -> (0:w258:bool)
            }
            n149 = local read "OK Input"() -> (w241:bool)
            n150 = Or Array Elements(Boolean array=w244) -> (logical OR=w242:bool)
            n151 = And(x=w241, y=w242) -> (x .and. y?=w240:bool)
            n152 = Not(x=w242) -> (.not. x?=w243:bool)
            n153 = And(x=w243, y=w241) -> (x .and. y?=w239:bool)
            n154 = case shown="True" w240 {
              frame False {
              }
              frame True {
                # "Identical channels"
                n155 = property on="Status" class="Str"("Text.TextColor"=u32 16711680 ("Text.Text Colors:Text Color"), "Value"="Identical camera channels! Please select different devices." ("Status")) -> ()  [unwired: 2 in, 2 out]
                n156 = property on="OK Input" class="Bool (strict)"("Value"=FALSE ("OK Button")) -> ()  [unwired: 2 in, 2 out]
              }
            }
            n157 = local write "CamInput"(w239) -> ()
            n158 = Select(t=SM_UserInterface."InitVideo", s=w239, f=w252) -> (s? t:f=w250:T7)
          }
          frame "InitVideo" {
            # "Properties"
            n159 = Wait (ms)(milliseconds to wait=u32 2000 ("millisecond multiple")) -> ()  [unwired: 1 out]
            n160 = property on="IMAQdxChannel 1" class="IMAQdx (strict)"("DisabledEnum"=T9."Disabled and Grayed Out" ("Disabled")) -> ()  [unwired: 2 in, 2 out]
            n161 = property on="IMAQdxChannel 2" class="IMAQdx (strict)"("DisabledEnum"=T9."Disabled and Grayed Out" ("Disabled")) -> ()  [unwired: 2 in, 2 out]
            n162 = property on="IMAQdxChannel 3" class="IMAQdx (strict)"("DisabledEnum"=T9."Disabled and Grayed Out" ("Disabled")) -> ()  [unwired: 2 in, 2 out]
            n163 = property on="IMAQdxChannel 4" class="IMAQdx (strict)"("DisabledEnum"=T9."Disabled and Grayed Out" ("Disabled")) -> ()  [unwired: 2 in, 2 out]
            n164 = property on="OK Input" class="Bool (strict)"("DisabledEnum"=T9."Disabled and Grayed Out" ("Disabled")) -> ()  [unwired: 2 in, 2 out]
            n165 = property on="Status" class="Str"("Text.TextColor"=u32 0 ("Text.Text Colors:Text Color"), "Value"="Initialisation of Video Acquisition" ("Status")) -> ()  [unwired: 2 in, 2 out]
          }
          frame "InitExpData" {
            # "Cam Stream"
            # "For image with \n1090x1020 px"
            # "User Input"
            # "Properties"
            n166 = Wait Until Next ms Multiple(millisecond multiple=u32 100) -> ()  [unwired: 1 out]
            n167 = property on="Folder" class="Path"("DisabledEnum"=T9."Enabled" ("Disabled")) -> ()  [unwired: 2 in, 2 out]
            n168 = property on="File Name" class="Str"("DisabledEnum"=T9."Enabled" ("Disabled")) -> ()  [unwired: 2 in, 2 out]
            n169 = property on="User" class="Str"("DisabledEnum"=T9."Enabled" ("Disabled")) -> ()  [unwired: 2 in, 2 out]
            n170 = property on="Bursting Mode" class="CmbBox"("DisabledEnum"=T9."Enabled" ("Disabled")) -> ()  [unwired: 2 in, 2 out]
            n171 = property on="Flow Rate Level" class="DigNum (strict)"("DisabledEnum"=T9."Enabled" ("Disabled")) -> ()  [unwired: 2 in, 2 out]
            n172 = property on="Experiment Infos" class="Str"("DisabledEnum"=T9."Enabled" ("Disabled")) -> ()  [unwired: 2 in, 2 out]
            n173 = property on="OK File" class="Bool (strict)"("DisabledEnum"=T9."Enabled" ("Disabled")) -> ()  [unwired: 2 in, 2 out]
            n174 = local write "Status"("Live Video ON" ("Status")) -> ()
            n175 = local read "Folder"() -> (w311:path)
            n176 = local read "File Name"() -> (w310:string)
            n177 = local read "User"() -> (w298:string)
            n178 = local read "Bursting Mode"() -> (w299:string)
            n179 = local read "Flow Rate Level"() -> (w296:i32)
            n180 = local read "Experiment Infos"() -> (w297:string)
            n181 = property on="Camera 1" class="ImageControl"("X Zoom"=-3 ("ZoomInteger:X Zoom"), "Y Zoom"=-3 ("ZoomInteger:Y Zoom"), "Zoom to Fit Mode"=FALSE, "Image Center X Position"=u32 960 ("Image Center Position:X Position"), "Image Center Y Position"=u32 510 ("Image Center Position:Y Position")) -> ()  [unwired: 2 in, 2 out]
            n182 = property on="Camera 2" class="ImageControl"("X Zoom"=-3 ("ZoomInteger:X Zoom"), "Y Zoom"=-3 ("ZoomInteger:Y Zoom"), "Zoom to Fit Mode"=FALSE, "Image Center X Position"=u32 960 ("Image Center Position:X Position"), "Image Center Y Position"=u32 510 ("Image Center Position:Y Position")) -> ()  [unwired: 2 in, 2 out]
            n183 = local write "Folder"(w311) -> ()
            n184 = local write "File Name"(w310) -> ()
            n185 = local write "User"(w298) -> ()
            n186 = local write "Bursting Mode"(w299) -> ()
            n187 = local write "Flow Rate Level"(w296) -> ()
            n188 = local write "Experiment Infos"(w297) -> ()
            n189 = local read "OK File"() -> (w308:bool)
            n190 = property on="Camera 3" class="ImageControl"("X Zoom"=-3 ("ZoomInteger:X Zoom"), "Y Zoom"=-3 ("ZoomInteger:Y Zoom"), "Zoom to Fit Mode"=FALSE, "Image Center X Position"=u32 960 ("Image Center Position:X Position"), "Image Center Y Position"=u32 510 ("Image Center Position:Y Position")) -> ()  [unwired: 2 in, 2 out]
            n191 = property on="Camera 4" class="ImageControl"("X Zoom"=-3 ("ZoomInteger:X Zoom"), "Y Zoom"=-3 ("ZoomInteger:Y Zoom"), "Zoom to Fit Mode"=FALSE, "Image Center X Position"=u32 960 ("Image Center Position:X Position"), "Image Center Y Position"=u32 510 ("Image Center Position:Y Position")) -> ()  [unwired: 2 in, 2 out]
            n192 = Select(t=SM_UserInterface."WaitRec", s=w308, f=w307) -> (s? t:f=w274:T7)
            n193 = flat-sequence {
              tunnel: [w314] -> w273
              tunnel: w274 -> [w314]
              frame #0 {
                n194 = Wait (ms)(milliseconds to wait=u32 500) -> ()  [unwired: 1 out]
              }
            }
          }
          frame "WaitRec" {
            # "Properties"
            n195 = Wait Until Next ms Multiple(millisecond multiple=u32 100) -> ()  [unwired: 1 out]
            n196 = property on="StartRecord" class="Bool (strict)"("DisabledEnum"=T9."Enabled" ("Disabled")) -> ()  [unwired: 2 in, 2 out]
            n197 = property on="Folder" class="Path"("DisabledEnum"=T9."Disabled and Grayed Out" ("Disabled")) -> ()  [unwired: 2 in, 2 out]
            n198 = property on="File Name" class="Str"("DisabledEnum"=T9."Disabled and Grayed Out" ("Disabled")) -> ()  [unwired: 2 in, 2 out]
            n199 = property on="User" class="Str"("DisabledEnum"=T9."Disabled and Grayed Out" ("Disabled")) -> ()  [unwired: 2 in, 2 out]
            n200 = property on="Bursting Mode" class="CmbBox"("DisabledEnum"=T9."Disabled and Grayed Out" ("Disabled")) -> ()  [unwired: 2 in, 2 out]
            n201 = property on="Experiment Infos" class="Str"("DisabledEnum"=T9."Disabled and Grayed Out" ("Disabled")) -> ()  [unwired: 2 in, 2 out]
            n202 = property on="OK File" class="Bool (strict)"("DisabledEnum"=T9."Disabled and Grayed Out" ("Disabled"), "Value"=FALSE ("OK Button File")) -> ()  [unwired: 2 in, 2 out]
            n203 = property on="Flow Rate Level" class="DigNum (strict)"("DisabledEnum"=T9."Disabled and Grayed Out" ("Disabled")) -> ()  [unwired: 2 in, 2 out]
            n204 = local read "StartRecord"() -> (w316:bool)
            n205 = Select(t=SM_UserInterface."Recording", s=w316, f=w317) -> (s? t:f=w328:T7)
          }
          frame "Recording" {
            # "Properties"
            n206 = Wait Until Next ms Multiple(millisecond multiple=u32 100) -> ()  [unwired: 1 out]
            n207 = property on="StartRecording" class="Bool (strict)"("DisabledEnum"=T9."Disabled and Grayed Out" ("Disabled")) -> ()  [unwired: 2 in, 2 out]
            n208 = property on="StopRecording" class="Bool (strict)"("DisabledEnum"=T9."Enabled" ("Disabled")) -> ()  [unwired: 2 in, 2 out]
            n209 = local write "Status"("Video Recording" ("Status")) -> ()
            n210 = local read "StopRecord"() -> (w334:bool)
            n211 = Select(t=SM_UserInterface."StopRec", s=w334, f=w336) -> (s? t:f=w335:T7)
          }
          frame "StopRec" {
            w343 = FALSE ("StopRecord")
            w345 = FALSE ("StopRecord")
            # "Properties"
            n212 = Wait Until Next ms Multiple(millisecond multiple=u32 100) -> ()  [unwired: 1 out]
            n213 = property on="StopRecord" class="Bool (strict)"("DisabledEnum"=T9."Disabled and Grayed Out" ("Disabled"), "Value"=w345, "Visible"=w345) -> ()  [unwired: 2 in, 2 out]
            n214 = property on="StartRecord" class="Bool (strict)"("DisabledEnum"=T9."Disabled and Grayed Out" ("Disabled"), "Value"=w343, "Visible"=w343) -> ()  [unwired: 2 in, 2 out]
            n215 = property on="Experiment Comment" class="Str"("DisabledEnum"=T9."Enabled" ("Disabled"), "Visible"=TRUE) -> ()  [unwired: 2 in, 2 out]
            n216 = property on="OK Exp" class="Bool (strict)"("DisabledEnum"=T9."Enabled" ("Disabled"), "Visible"=TRUE) -> ()  [unwired: 2 in, 2 out]
          }
          frame Default {
          }
        }
        n217 = Tick Count (ms)() -> (millisecond timer value=w236:u32)
        n218 = feedback #1(u32 0 ("millisecond timer value")) -> (w237:u32)
        n219 = feedback-in #1(w236) -> ()
        n220 = Subtract(x=w236, y=w237) -> (x-y=w233:u32)
        n221 = local write "LoopTimer UI"(w233) -> ()
        n222 = local write "StateUI"(w234) -> ()
        n223 = local read "Stop"() -> (w232:bool)
      }
      n224 = timed-loop {
        timing: w139 -> [_]
        timing-out: [_] -> w138
        shift-right: [w348] -> _
        shift-left: _ -> [w365]
        tunnel: w126 -> [w362]
        tunnel: [w361] -> w135
        tunnel: [w355] -> w137
        tunnel: [w360] -> w136
        tunnel: [w359] -> w134
        tunnel: w126 -> [w352]
        stop <- w356 stop-if-true
        # "No error"
        # "Filter"
        # "AMSYS AMS5812 0050-D\nResolution: 0.129 mmHg\nAccuracy: 1.29 mmHg\n->Output resolution 0.1 mmHg"
        # "Resolution 0.5°C \nAccuracy 0.5°C"
        # "Sensor Data Acquisition (Sensor Producer)"
        n225 = node-c288() -> ()  [unwired: 1 in, 1 out]
        n226 = shared-variable "NI-myRIO-1900-Biomech\\myRIO_Data.lvlib\\RawData_PressureSensor"(error in=w362) -> (w367:u8[], error out=w355:errorcluster)  [unwired: 1 out]
        n227 = shared-variable "NI-myRIO-1900-Biomech\\myRIO_Data.lvlib\\RawData_TempSensor"(error in=w352) -> (w368:u8[], error out=w349:errorcluster)  [unwired: 1 out]
        n228 = call "AMS5812_Convert Raw Pressure Temp.vi"("Read Data"=w367) -> ("Pressure rounded (mmHg)"=w366:dbl, "Temp (C)"=w364:dbl)  [unwired: 5 in, 4 out]
        n229 = Unbundle(w355) -> ("status"=w353:bool)  [unwired: 2 out]
        n230 = call "DS18B20_Convert Raw Temp.vi"("Scratchpad Data"=w368) -> ("Temp rounded (C)"=w363:dbl)  [unwired: 6 in, 2 out]
        n231 = Unbundle(w349) -> ("status"=w351:bool)  [unwired: 2 out]
        n232 = Not(x=w353) -> (.not. x?=w354:bool)
        n233 = Not(x=w351) -> (.not. x?=w350:bool)
        n234 = local write "Status Pressure Sensor"(w354) -> ()
        n235 = local write "Status Temp. Sensor"(w350) -> ()
        n236 = Greater?(x=w366, y=260.0) -> (0:w357:bool)
        n237 = Select(t=w365, s=w357, f=w366) -> (s? t:f=w348:dbl)
        n238 = shared-variable ".\\Data Buffer.lvlib\\Pressure Buffer"(w348, error in=w355) -> (error out=w360:errorcluster)
        n239 = shared-variable ".\\Data Buffer.lvlib\\Pressure Temp Buffer"(w364, error in=w355) -> (error out=w361:errorcluster)
        n240 = shared-variable ".\\Data Buffer.lvlib\\Temp Buffer"(w363, error in=w349) -> (error out=w359:errorcluster)
        n241 = local read "Stop"() -> (w356:bool)
        n242 = node-c288() -> ()  [unwired: 1 in, 1 out]
      }
      n243 = while {
        shift-right: [w377] -> _
        shift-left: w140 -> [w373]
        shift-right: [w380] -> _
        shift-left: _ -> [w378]
        shift-right: [w379] -> _
        shift-left: _ -> [w376]
        i -> [w374]
        stop <- w375 stop-if-true
        # "Sensor Data Log (Sensor Consumer)"
        n244 = case shown="\"FirstCallWriteData\"" w373 {
          selector: w373 -> [w386 w402 w469 w478 _ w527 w584 w601 w609]
          tunnel: [w387 w403 w470 w479 SM_DataLog."WriteData" w529 w587 w601 w609] -> w377
          tunnel: [w385 w399 w460 w477 w525 w538 w590 w599 w610] -> w380
          tunnel: [w381 w400 w467 w476 w526 w537 w591 w603 w611] -> w379
          tunnel: w378 -> [w385 w399 _ w477 w496 w536 w588 w599 w610]
          tunnel: w376 -> [w381 w411 w459 w476 w495 w534 w589 w602 w611]
          frame "Wait" {
            n245 = Wait Until Next ms Multiple(millisecond multiple=u32 100 ("millisecond timer value")) -> ()  [unwired: 1 out]
            n246 = local read "OK File"() -> (w382:bool)
            n247 = Select(t=SM_DataLog."CreateFolder", s=w382, f=w386) -> (s? t:f=w387:T6)
          }
          frame "CreateFolder" {
            # "Start Time for Create Folder & Files"
            # "Folder"
            # "Name: YYYYMMDD-HHMM-Filename"
            n248 = Get Date/Time In Seconds() -> (seconds since 1Jan1904=w418:timestamp)
            n249 = Wait Until Next ms Multiple(millisecond multiple=u32 500 ("millisecond timer value")) -> ()  [unwired: 1 out]
            n250 = Format Date/Time String(time format string (%c)="%d.%m.20%y", seconds (now)=w418) -> (date/time string=w413:string)  [unwired: 1 in]
            n251 = Format Date/Time String(time format string (%c)="%H:%M:%S", seconds (now)=w418) -> (date/time string=w412:string)  [unwired: 1 in]
            n252 = Format Date/Time String(time format string (%c)="20%y%m%d-%H%M%S-", seconds (now)=w418) -> (date/time string=w417:string)  [unwired: 1 in]
            n253 = local write "Start_DateTime"(w417) -> ()
            n254 = flat-sequence {
              tunnel: w411 -> [w449]
              tunnel: [w449] -> w410
              tunnel: [w447] -> w389
              tunnel: [w446] -> w388
              frame #0 {
                # "Data folder"
                n255 = Wait (ms)(milliseconds to wait=u32 200) -> ()  [unwired: 1 out]
                n256 = local read "File Name"() -> (w446:string)
                n257 = local read "Folder"() -> (w447:path)
              }
            }
            n258 = Match Pattern(string=w412, regular expression=":" ("string"), offset (0)=2) -> (before substring=w439:string, after substring=w441:string)  [unwired: 2 out]
            n259 = Match Pattern(string=w413, regular expression=".", offset (0)=2) -> (before substring=w421:string, after substring=w440:string)  [unwired: 2 out]
            n260 = Match Pattern(string=w440, regular expression=".", offset (0)=2) -> (before substring=w420:string, after substring=w419:string)  [unwired: 2 out]
            n261 = Match Pattern(string=w441, regular expression=":", offset (0)=2) -> (before substring=w438:string, after substring=w422:string)  [unwired: 2 out]
            n262 = Match Pattern(string=w422, regular expression=":", offset (0)=2) -> (before substring=w423:string)  [unwired: 3 out]
            n263 = Format Into String(format string="%s%s%s%s%s%s%s%s%s", w419, w420, w421, "-" ("regular expression"), w439, w438, w423, "-" ("regular expression"), w388) -> (resulting string=w392:string)  [unwired: 2 in, 1 out]
            n264 = Build Path(base path=w389, name or relative path=w392) -> (appended path=w407:path)
            n265 = Create Folder(path (use dialog)=w407, error in=w410) -> (created path=w426:path, error out=w393:errorcluster)  [unwired: 1 in, 1 out]
            n266 = flat-sequence {
              tunnel: [w444] -> w394
              tunnel: w393 -> [w444]
              tunnel: w392 -> [w443]
              tunnel: [w443] -> w391
              tunnel: [w442] -> w390
              tunnel: w389 -> [w442]
              frame #0 {
                n267 = Wait (ms)(milliseconds to wait=u32 200) -> ()  [unwired: 1 out]
              }
            }
            n268 = local write "LogFolder"(w426) -> ()
            n269 = List Folder(path=w390, error in=w394) -> (folder names=w406:string[], error out=w400:errorcluster)  [unwired: 2 in, 2 out]
            n270 = Search 1D Array(1D array=w406, element=w391, start index (0)=0) -> (index of element=w405:i32)
            n271 = Equal?(x=w405, y=-1) -> (x = y?=w397:bool)
            n272 = Select(t="No folder could be created" ("Status"), s=w397, f="Create Folder") -> (s? t:f=w396:string)
            n273 = local write "Status"(w396) -> ()
            n274 = Select(t=w402, s=w397, f=SM_DataLog."CreateFile") -> (s? t:f=w403:T6)
          }
          frame "CreateFile" {
            # "Created File?"
            # "File"
            n275 = Wait Until Next ms Multiple(millisecond multiple=u32 500 ("millisecond timer value")) -> ()  [unwired: 1 out]
            n276 = local read "LogFolder"() -> (w455:path)
            n277 = local read "File Name"() -> (w466:string)
            n278 = Format Into String(format string="%s%s", w466, ".txt" ("string")) -> (resulting string=w456:string)  [unwired: 2 in, 1 out]
            n279 = Build Path(base path=w455, name or relative path=w456) -> (appended path=w465:path)
            n280 = Open/Create/Replace File(file path (use dialog)=w465, error in=w459, operation (0:open)=T13."create", access (0:read/write)=enum16{"read/write", "read-only", "write-only"}."read/write") -> (refnum out=w460:refnum<file>, error out=w458:errorcluster)  [unwired: 2 in, 1 out]
            n281 = List Folder(path=w455, error in=w458) -> (filenames=w457:string[], error out=w467:errorcluster)  [unwired: 2 in, 2 out]
            n282 = Search 1D Array(1D array=w457, element=w456, start index (0)=0) -> (index of element=w472:i32)
            n283 = Equal?(x=w472, y=-1) -> (x = y?=w450:bool)
            n284 = Not(x=w450) -> (.not. x?=w454:bool)
            n285 = Select(t="No file could be created" ("Status"), s=w450, f="Create File") -> (s? t:f=w453:string)
            n286 = local write "DataFile"(w454) -> ()
            n287 = local write "Status"(w453) -> ()
            n288 = Select(t=w469, s=w450, f=SM_DataLog."WaitRec") -> (s? t:f=w470:T6)
          }
          frame "WaitRec" {
            n289 = Wait Until Next ms Multiple(millisecond multiple=u32 100) -> ()  [unwired: 1 out]
            n290 = local read "StartRecord"() -> (w481:bool)
            n291 = Select(t=SM_DataLog."FirstCallWriteData" ("SM_DataLog"), s=w481, f=w478) -> (s? t:f=w479:T6)
            n292 = local write "Status"("Live Video ON" ("Status")) -> ()
          }
          frame "FirstCallWriteData" {
            w490 = 0 ("PrevActualTime_ms")
            # "StartTime"
            # "StartDate"
            # "First Input"
            # "Header"
            # "Start Time"
            # "StartTime"
            # "StartDate"
            # "Start Pressure"
            n293 = Get Date/Time In Seconds() -> (seconds since 1Jan1904=w491:timestamp)
            n294 = property on="Cam1 Time" class="Str"("Visible"=TRUE) -> ()  [unwired: 2 in, 2 out]
            n295 = property on="Cam2 Time" class="Str"("Visible"=TRUE) -> ()  [unwired: 2 in, 2 out]
            n296 = property on="Cam3 Time" class="Str"("Visible"=TRUE) -> ()  [unwired: 2 in, 2 out]
            n297 = property on="Cam4 Time" class="Str"("Visible"=TRUE) -> ()  [unwired: 2 in, 2 out]
            n298 = call "ExpTimeConversion.vi"("PrevExpTime_ms"=w490, "PrevActualTime_ms"=w490, "time stamp"=w491) -> ("ActualTime_ms"=w492:i32, "ActualTimeString"=w488:string, "ActualDateString"=w489:string)  [unwired: 5 in, 1 out]
            n299 = local write "ActualTime_ms"(w492) -> ()
            n300 = local write "ExpTime_ms"(w490) -> ()
            n301 = local read "User"() -> (w503:string)
            n302 = local read "Bursting Mode"() -> (w501:string)
            n303 = local read "Flow Rate Level"() -> (w498:i32)
            n304 = local read "Experiment Infos"() -> (w502:string)
            n305 = local read "Pressure (mmHg)"() -> (w499:dbl)
            n306 = local read "File Name"() -> (w487:string)
            n307 = local write "StartPressure (mmHg)"(w499) -> ()
            n308 = Number To Fractional String(number=w499, precision (6)=i16 3) -> (F-format string=w500:string)  [unwired: 2 in]
            n309 = call "DataRecording_Header.vi"("User"=w503, "StartDate"=w489, "StartTime"=w488, "Bursting Mode"=w501, "Flow Rate Level"=w498, "Experiment Infos"=w502, "Test Name"=w487, "StartPressure"=w500) -> ("Header"=w504:string)  [unwired: 11 in]
            n310 = Write to Text File(file (use dialog)=w496, text=w504, error in=w495) -> (refnum out=w494:refnum<file>, error out=w493:errorcluster)  [unwired: 1 in, 1 out]
            n311 = local read "Temp (C)"() -> (w520:dbl)
            n312 = local read "Pressure (mmHg)"() -> (w515:dbl)
            n313 = local read "Pressure Temp (C)"() -> (w511:dbl)
            n314 = Number To Fractional String(number=w520, precision (6)=i16 1) -> (F-format string=w518:string)  [unwired: 2 in]
            n315 = Number To Fractional String(number=w515, precision (6)=i16 2) -> (F-format string=w514:string)  [unwired: 2 in]
            n316 = Number To Fractional String(number=w511, precision (6)=i16 1) -> (F-format string=w510:string)  [unwired: 2 in]
            n317 = Concatenate Strings(w489, ";", w488, ";", "0;", w518, ";", w514, ";", "0;", "0;", w510, ";", "\r\n") -> (w524:string)
            n318 = Write to Text File(file (use dialog)=w494, text=w524, error in=w493) -> (refnum out=w525:refnum<file>, error out=w526:errorcluster)  [unwired: 1 in, 1 out]
          }
          frame "WriteData" {
            # "Write Time"
            n319 = flat-sequence {
              tunnel: [w542] -> w532
              tunnel: [w541] -> w531
              tunnel: [w540] -> w530
              tunnel: [w539] -> w528
              tunnel: w527 -> [w539]
              tunnel: [w566] -> w533
              tunnel: w532 -> [w555]
              tunnel: w531 -> [w554]
              tunnel: w530 -> [w553]
              tunnel: [w550] -> w529
              tunnel: w528 -> [w549]
              frame #0 {
                # "ActualTime String"
                # "ActualDateString"
                # "Time stamp display"
                # "Timer"
                n320 = Get Date/Time In Seconds() -> (seconds since 1Jan1904=w544:timestamp)
                n321 = local read "ActualTime_ms"() -> (w548:i32)
                n322 = local read "ExpTime_ms"() -> (w547:i32)
                n323 = Format Date/Time String(time format string (%c)="%H:%M:%S%3u", seconds (now)=w544) -> (date/time string=w543:string)  [unwired: 1 in]
                n324 = call "ExpTimeConversion.vi"("PrevExpTime_ms"=w547, "PrevActualTime_ms"=w548, "time stamp"=w544) -> ("ExpTime_ms"=w540:i32, "ActualTime_ms"=w546:i32, "ActualTimeString"=w541:string, "ActualDateString"=w542:string)  [unwired: 5 in]
                n325 = local write "Cam1 Time"(w543) -> ()
                n326 = local write "Cam2 Time"(w543) -> ()
                n327 = local write "Cam3 Time"(w543) -> ()
                n328 = local write "Cam4 Time"(w543) -> ()
                n329 = local write "ActualTime_ms"(w546) -> ()
                n330 = local write "ExpTime_ms"(w540) -> ()
              }
              frame #1 {
                n331 = local read "Temp (C)"() -> (w577:dbl)
                n332 = local read "Pressure (mmHg)"() -> (w563:dbl)
                n333 = local read "StartPressure (mmHg)"() -> (w564:dbl)
                n334 = local read "meanPressure"() -> (w558:dbl)
                n335 = local read "Pressure Temp (C)"() -> (w580:dbl)
                n336 = Number To Decimal String(number=w553) -> (decimal integer string=w582:string)  [unwired: 1 in]
                n337 = local read "StartRecord"() -> (w552:bool)
                n338 = Subtract(x=w563, y=w564) -> (x-y=w561:dbl)
                n339 = Number To Fractional String(number=w577, precision (6)=i16 1) -> (F-format string=w578:string)  [unwired: 2 in]
                n340 = Number To Fractional String(number=w563, precision (6)=i16 2) -> (F-format string=w579:string)  [unwired: 2 in]
                n341 = Number To Fractional String(number=w561, precision (6)=i16 2) -> (F-format string=w560:string)  [unwired: 2 in]
                n342 = Number To Fractional String(number=w558, precision (6)=i16 2) -> (F-format string=w557:string)  [unwired: 2 in]
                n343 = Number To Fractional String(number=w580, precision (6)=i16 1) -> (F-format string=w581:string)  [unwired: 2 in]
                n344 = Select(t=w549, s=w552, f=SM_DataLog."LastCallWriteData") -> (s? t:f=w550:T6)
                n345 = Concatenate Strings(w555, ";", w554, ";", w582, ";", w578, ";", w579, ";", w560, ";", w557, ";", w581, ";", "\r\n") -> (w566:string)
              }
            }
            n346 = Wait Until Next ms Multiple(millisecond multiple=u32 100 ("millisecond timer value")) -> ()  [unwired: 1 out]
            n347 = Write to Text File(file (use dialog)=w536, text=w533, error in=w534) -> (refnum out=w538:refnum<file>, error out=w537:errorcluster)  [unwired: 1 in, 1 out]
          }
          frame "LastCallWriteData" {
            n348 = Wait Until Next ms Multiple(millisecond multiple=u32 100 ("millisecond timer value")) -> ()  [unwired: 1 out]
            n349 = local read "OK Exp"() -> (w586:bool)
            n350 = Select(t=SM_DataLog."Stop", s=w586, f=w584) -> (s? t:f=w587:T6)
            n351 = case shown="True" w586 {
              tunnel: [w592 w598] -> w591
              tunnel: [w593 w597] -> w590
              tunnel: w589 -> [w592 w596]
              tunnel: w588 -> [w593 w595]
              frame False {
              }
              frame True {
                n352 = local read "Experiment Comment"() -> (w594:string)
                n353 = Write to Text File(file (use dialog)=w595, text=w594, error in=w596) -> (refnum out=w597:refnum<file>, error out=w598:errorcluster)  [unwired: 1 in, 1 out]
              }
            }
          }
          frame "Stop" {
            n354 = flat-sequence {
              tunnel: w599 -> [w605]
              tunnel: w602 -> [w604]
              tunnel: [w606] -> w600
              tunnel: [w608] -> w603
              tunnel: w600 -> [w608]
              frame #0 {
                n355 = Close File(refnum=w605, error in=w604) -> (error out=w606:errorcluster)  [unwired: 1 out]
              }
              frame #1 {
                n356 = local write "Cancel"(TRUE ("Cancel")) -> ()
              }
            }
          }
          frame Default {
          }
        }
        n357 = local write "IncLoop DataLog"(w374) -> ()
        n358 = local write "StateDataLog"(w377) -> ()
        n359 = local read "Stop"() -> (w375:bool)
      }
      n360 = while {
        tunnel: w127 -> [w226]
        shift-right: [w222] -> _
        shift-left: w128 -> [w229]
        tunnel: [w224] -> _
        stop <- w225 stop-if-true
        # "Smoothing Filter"
        # "Array with last 20 values"
        # "Fills array"
        # "Sensor Mean (Sensor Consumer)"
        n361 = Wait (ms)(milliseconds to wait=u32 100 ("millisecond multiple")) -> ()  [unwired: 1 out]
        n362 = shared-variable ".\\Data Buffer.lvlib\\Pressure Buffer"() -> (w230:dbl, error out=w224:errorcluster)  [unwired: 1 in]
        n363 = Insert Into Array(array=w229, index=0, new element=w230) -> (w227:dbl[])
        n364 = Array Subset(array=w227, length=w226) -> (w222:dbl[])  [unwired: 1 in]
        n365 = call-poly <vilib>:"Mean.vi"("X"=w222) -> ("mean"=w223:dbl)  [unwired: 1 out]
        n366 = local write "meanPressureArray"(w222) -> ()
        n367 = local write "meanPressure"(w223) -> ()
        n368 = local read "Stop"() -> (w225:bool)
      }
      n369 = while {
        tunnel: [w630] -> w131
        tunnel: [w629] -> w132
        tunnel: [w628] -> w133
        stop <- w625 stop-if-true
        w643 = 1.0 ("y")
        w648 = 1.0 ("y")
        w613 = 0.2 ("dt")
        # "AMSYS AMS5812 0030-D\nResolution: 0,0775 mmHg\nAccuracy: 0,775 mmHg\n->Output resolution 0,05 mmHg"
        # "Dynamic scale of axes"
        # "Dynamic scale of axes"
        # "x-axis time"
        # "x-axis time"
        # "seconds \n(loop time)"
        # "seconds \n(loop time)"
        # "Resolution 0.5°C \nAccuracy 0.5°C"
        # "Sensor User Interface (Sensor Consumer)"
        n370 = shared-variable ".\\Data Buffer.lvlib\\Pressure Buffer"() -> (w624:dbl, error out=w630:errorcluster)  [unwired: 1 in]
        n371 = shared-variable ".\\Data Buffer.lvlib\\Pressure Temp Buffer"() -> (w632:dbl, error out=w629:errorcluster)  [unwired: 1 in]
        n372 = shared-variable ".\\Data Buffer.lvlib\\Temp Buffer"() -> (w631:dbl, error out=w628:errorcluster)  [unwired: 1 in]
        n373 = Wait (ms)(milliseconds to wait=u32 200 ("millisecond multiple")) -> ()  [unwired: 1 out]
        n374 = local read "meanPressure"() -> (w623:dbl)
        n375 = local write "Pressure (mmHg)"(w624) -> ()
        n376 = local write "Temp (C)"(w631) -> ()
        n377 = local write "Pressure Temp (C)"(w632) -> ()
        n378 = Get Date/Time In Seconds() -> (seconds since 1Jan1904=w612:timestamp)
        n379 = Build Array(w624) -> (w614:dbl[])
        n380 = Build Array(w623) -> (w616:dbl[])
        n381 = Build Array(w631) -> (w652:dbl[])
        n382 = Get Date/Time In Seconds() -> (seconds since 1Jan1904=w637:timestamp)
        n383 = Bundle By Name("Y"=w652, "dt"=0.2, "t0"=w637) -> (w645:waveform(dbl))  [unwired: 1 in]
        n384 = Bundle By Name("Y"=w614, "dt"=w613, "t0"=w612) -> (w622:waveform(dbl))  [unwired: 1 in]
        n385 = Bundle By Name("dt"=w613, "t0"=w612, "Y"=w616) -> (w621:waveform(dbl))  [unwired: 1 in]
        n386 = local write "Waveform Chart Temp"(w645) -> ()
        n387 = Build Array(w622, w621) -> (w615:waveform(dbl)[])
        n388 = local write "Waveform Pressure Cluster"(w615) -> ()
        n389 = Unbundle By Name(w622) -> ("Y"=w644:dbl[])
        n390 = Unbundle By Name(w645) -> ("Y"=w647:dbl[])
        n391 = To Double Precision Float(number=w612) -> (double precision float=w617:dbl)
        n392 = Index Array(array=w644) -> (element=w640:dbl)  [unwired: 1 in]
        n393 = To Double Precision Float(number=w637) -> (double precision float=w634:dbl)
        n394 = Index Array(array=w647) -> (element=w646:dbl)  [unwired: 1 in]
        n395 = call <vilib>:"Array Max & Min PtByPt.vi"("input data point"=w640, "sample length"=50) -> ("max value"=w641:dbl, "min value"=w642:dbl)  [unwired: 1 in, 3 out]
        n396 = call <vilib>:"Array Max & Min PtByPt.vi"("input data point"=w646, "sample length"=50) -> ("max value"=w651:dbl, "min value"=w649:dbl)  [unwired: 1 in, 3 out]
        n397 = Add(x=w641, y=w643) -> (x+y=w620:dbl)
        n398 = Subtract(x=w642, y=w643) -> (x-y=w619:dbl)
        n399 = Subtract(x=w617, y=10.0) -> (x-y=w618:dbl)
        n400 = Add(x=w651, y=w648) -> (x+y=w650:dbl)
        n401 = Subtract(x=w649, y=w648) -> (x-y=w639:dbl)
        n402 = Subtract(x=w634, y=10.0) -> (x-y=w635:dbl)
        n403 = property on="Waveform Pressure Cluster" class="WFChart (strict)"("YScale.Maximum"=w620, "YScale.Minimum"=w619, "XScale.Minimum"=w618, "XScale.Maximum"=w617) -> ()  [unwired: 2 in, 2 out]
        n404 = property on="Waveform Chart Temp" class="WFChart (strict)"("YScale.Maximum"=w650, "YScale.Minimum"=w639, "XScale.Minimum"=w635, "XScale.Maximum"=w634) -> ()  [unwired: 2 in, 2 out]
        n405 = local read "Stop"() -> (w625:bool)
      }
      n406 = while {
        stop <- w220 stop-if-true
        # "Global stop"
        # "Cancel FrontPanel = Cancel Exp./VI and stops all Loops\nOK Exp. = Experiment completed \n-> write last comment to storage file -> Set cancel true"
        # "Stop"
        n407 = Wait Until Next ms Multiple(millisecond multiple=u32 50) -> ()  [unwired: 1 out]
        n408 = local read "Cancel"() -> (w220:bool)
        n409 = local write "Stop"(w220) -> ()
      }
      n410 = while {
        stop <- w186 stop-if-true
        # "Developer"
        n411 = local read "Developer"() -> (w184:bool)
        n412 = Wait Until Next ms Multiple(millisecond multiple=u32 100) -> ()  [unwired: 1 out]
        n413 = case shown="True" w184 {
          frame True {
            w190 = TRUE ("Visible")
            w188 = TRUE ("Visible")
            w189 = TRUE ("Visible")
            w187 = TRUE ("Visible")
            w196 = TRUE ("Visible")
            w195 = TRUE ("Visible")
            w194 = TRUE ("Visible")
            w192 = TRUE ("Visible")
            w193 = TRUE ("Visible")
            n414 = property on="LoopTimer Cam3" class="Clust (strict)"("Visible"=w189) -> ()  [unwired: 2 in, 2 out]
            n415 = property on="WriteSpeed Cam3" class="Clust (strict)"("Visible"=w189) -> ()  [unwired: 2 in, 2 out]
            n416 = property on="Frames Cam3" class="Clust (strict)"("Visible"=w189) -> ()  [unwired: 2 in, 2 out]
            n417 = property on="Buffer Cam3" class="Clust (strict)"("Visible"=w189) -> ()  [unwired: 2 in, 2 out]
            n418 = property on="LoopTimer Cam1" class="Clust (strict)"("Visible"=w187) -> ()  [unwired: 2 in, 2 out]
            n419 = property on="WriteSpeed Cam1" class="Clust (strict)"("Visible"=w187) -> ()  [unwired: 2 in, 2 out]
            n420 = property on="Frames Cam1" class="Clust (strict)"("Visible"=w187) -> ()  [unwired: 2 in, 2 out]
            n421 = property on="Buffer Cam1" class="Clust (strict)"("Visible"=w187) -> ()  [unwired: 2 in, 2 out]
            n422 = property on="error out" class="Clust (strict)"("Visible"=TRUE) -> ()  [unwired: 2 in, 2 out]
            n423 = property on="StateUI" class="Enum (strict)"("Visible"=w195) -> ()  [unwired: 2 in, 2 out]
            n424 = property on="LoopTimer UI" class="DigNum (strict)"("Visible"=w195) -> ()  [unwired: 2 in, 2 out]
            n425 = property on="Pressure Temp (C)" class="DigNum (strict)"("Visible"=w193) -> ()  [unwired: 2 in, 2 out]
            n426 = property on="StartPressure (mmHg)" class="DigNum (strict)"("Visible"=w193) -> ()  [unwired: 2 in, 2 out]
            n427 = property on="meanPressure" class="DigNum (strict)"("Visible"=w193) -> ()  [unwired: 2 in, 2 out]
            n428 = property on="meanPressureArray" class="Arr (strict)"("Visible"=w193) -> ()  [unwired: 2 in, 2 out]
            n429 = property on="LoopTimer Cam2" class="Clust (strict)"("Visible"=w188) -> ()  [unwired: 2 in, 2 out]
            n430 = property on="WriteSpeed Cam2" class="Clust (strict)"("Visible"=w188) -> ()  [unwired: 2 in, 2 out]
            n431 = property on="Frames Cam2" class="Clust (strict)"("Visible"=w188) -> ()  [unwired: 2 in, 2 out]
            n432 = property on="Buffer Cam2" class="Clust (strict)"("Visible"=w188) -> ()  [unwired: 2 in, 2 out]
            n433 = property on="LoopTimer Cam4" class="Clust (strict)"("Visible"=w190) -> ()  [unwired: 2 in, 2 out]
            n434 = property on="WriteSpeed Cam4" class="Clust (strict)"("Visible"=w190) -> ()  [unwired: 2 in, 2 out]
            n435 = property on="Frames Cam4" class="Clust (strict)"("Visible"=w190) -> ()  [unwired: 2 in, 2 out]
            n436 = property on="Buffer Cam4" class="Clust (strict)"("Visible"=w190) -> ()  [unwired: 2 in, 2 out]
            n437 = property on="LogFolder" class="Path"("Visible"=w194) -> ()  [unwired: 2 in, 2 out]
            n438 = property on="CamInput" class="Bool (strict)"("Visible"=w194) -> ()  [unwired: 2 in, 2 out]
            n439 = property on="StateDataLog" class="Enum (strict)"("Visible"=w196) -> ()  [unwired: 2 in, 2 out]
            n440 = property on="IncLoop DataLog" class="DigNum (strict)"("Visible"=w196) -> ()  [unwired: 2 in, 2 out]
            n441 = property on="ActualTime_ms" class="DigNum (strict)"("Visible"=w192) -> ()  [unwired: 2 in, 2 out]
            n442 = property on="ExpTime_ms" class="DigNum (strict)"("Visible"=w192) -> ()  [unwired: 2 in, 2 out]
            n443 = property on="Start_DateTime" class="Str"("Visible"=w192) -> ()  [unwired: 2 in, 2 out]
          }
          frame False {
            w197 = FALSE ("Visible")
            w199 = FALSE ("Visible")
            w198 = FALSE ("Visible")
            w200 = FALSE ("Visible")
            w206 = FALSE ("Visible")
            w205 = FALSE ("Visible")
            w204 = FALSE ("Visible")
            w202 = FALSE ("Visible")
            w203 = FALSE ("Visible")
            n444 = property on="LoopTimer Cam3" class="Clust (strict)"("Visible"=w198) -> ()  [unwired: 2 in, 2 out]
            n445 = property on="WriteSpeed Cam3" class="Clust (strict)"("Visible"=w198) -> ()  [unwired: 2 in, 2 out]
            n446 = property on="Frames Cam3" class="Clust (strict)"("Visible"=w198) -> ()  [unwired: 2 in, 2 out]
            n447 = property on="Buffer Cam3" class="Clust (strict)"("Visible"=w198) -> ()  [unwired: 2 in, 2 out]
            n448 = property on="error out" class="Clust (strict)"("Visible"=FALSE) -> ()  [unwired: 2 in, 2 out]
            n449 = property on="StateUI" class="Enum (strict)"("Visible"=w205) -> ()  [unwired: 2 in, 2 out]
            n450 = property on="LoopTimer UI" class="DigNum (strict)"("Visible"=w205) -> ()  [unwired: 2 in, 2 out]
            n451 = property on="Pressure Temp (C)" class="DigNum (strict)"("Visible"=w203) -> ()  [unwired: 2 in, 2 out]
            n452 = property on="StartPressure (mmHg)" class="DigNum (strict)"("Visible"=w203) -> ()  [unwired: 2 in, 2 out]
            n453 = property on="meanPressure" class="DigNum (strict)"("Visible"=w203) -> ()  [unwired: 2 in, 2 out]
            n454 = property on="meanPressureArray" class="Arr (strict)"("Visible"=w203) -> ()  [unwired: 2 in, 2 out]
            n455 = property on="LoopTimer Cam1" class="Clust (strict)"("Visible"=w200) -> ()  [unwired: 2 in, 2 out]
            n456 = property on="WriteSpeed Cam1" class="Clust (strict)"("Visible"=w200) -> ()  [unwired: 2 in, 2 out]
            n457 = property on="Frames Cam1" class="Clust (strict)"("Visible"=w200) -> ()  [unwired: 2 in, 2 out]
            n458 = property on="Buffer Cam1" class="Clust (strict)"("Visible"=w200) -> ()  [unwired: 2 in, 2 out]
            n459 = property on="LoopTimer Cam2" class="Clust (strict)"("Visible"=w199) -> ()  [unwired: 2 in, 2 out]
            n460 = property on="WriteSpeed Cam2" class="Clust (strict)"("Visible"=w199) -> ()  [unwired: 2 in, 2 out]
            n461 = property on="Frames Cam2" class="Clust (strict)"("Visible"=w199) -> ()  [unwired: 2 in, 2 out]
            n462 = property on="Buffer Cam2" class="Clust (strict)"("Visible"=w199) -> ()  [unwired: 2 in, 2 out]
            n463 = property on="LoopTimer Cam4" class="Clust (strict)"("Visible"=w197) -> ()  [unwired: 2 in, 2 out]
            n464 = property on="WriteSpeed Cam4" class="Clust (strict)"("Visible"=w197) -> ()  [unwired: 2 in, 2 out]
            n465 = property on="Frames Cam4" class="Clust (strict)"("Visible"=w197) -> ()  [unwired: 2 in, 2 out]
            n466 = property on="Buffer Cam4" class="Clust (strict)"("Visible"=w197) -> ()  [unwired: 2 in, 2 out]
            n467 = property on="LogFolder" class="Path"("Visible"=w204) -> ()  [unwired: 2 in, 2 out]
            n468 = property on="CamInput" class="Bool (strict)"("Visible"=w204) -> ()  [unwired: 2 in, 2 out]
            n469 = property on="StateDataLog" class="Enum (strict)"("Visible"=w206) -> ()  [unwired: 2 in, 2 out]
            n470 = property on="IncLoop DataLog" class="DigNum (strict)"("Visible"=w206) -> ()  [unwired: 2 in, 2 out]
            n471 = property on="ActualTime_ms" class="DigNum (strict)"("Visible"=w202) -> ()  [unwired: 2 in, 2 out]
            n472 = property on="ExpTime_ms" class="DigNum (strict)"("Visible"=w202) -> ()  [unwired: 2 in, 2 out]
            n473 = property on="Start_DateTime" class="Str"("Visible"=w202) -> ()  [unwired: 2 in, 2 out]
          }
        }
        n474 = local read "Stop"() -> (w186:bool)
      }
      n475 = node-c288(w138) -> ()  [unwired: 1 out]
      n476 = disable-structure shown="Disabled" {
        frame Disabled {
          # "Alternative Filter"
          n477 = call "Convert to Dynamic Data"() -> ("Dynamic Data Type"=w143:dynamicdata)  [unwired: 4 in]
          n478 = call "Filter"("Signal"=w143) -> ("Filtered Signal"=w144:dynamicdata)  [unwired: 9 in, 1 out]
          n479 = call "Convert from Dynamic Data"("Dynamic Data Type"=w144) -> ()  [unwired: 3 in, 1 out]
        }
        frame Enabled {
        }
      }
    }
    frame #3 {
      # "Close Reference"
      # "Reset"
      n480 = Close Reference(reference=w663, error in (no error)=w660) -> (error out=w665:errorcluster)
      n481 = Close Reference(reference=w664, error in (no error)=w665) -> (error out=w662:errorcluster)
      n482 = Merge Errors(w662, w659, w658, w657, w654, w655, w656) -> (w661:errorcluster)
      n483 = local write "error out"(w661) -> ()
    }
  }
